vi "EventStream-GetPhotonInfo.vi"() -> ()   [LabVIEW 2023]
doc: "This example demonstrates how to use the Becker&Hickl LabVIEW wrapper VIs to acquire a decay curve using the FIFO Stream mode.\nA measurement is stopped either when accumulating the desired number of photons or the collection time expired.\nThe SPC parameters can be adjusted during the run. The rates and status flags are continuously updated.\nThis VI is based on the C-example part 5 in use_spcm.c\n\ninfo@becker-hickl.com"
uses:
  SPC_Wrappers/SPC_Controls/Fifo_Type.ctl
  SPC_Wrappers/SPC_Controls/SPC_RatesCluster.ctl
  Example_Controls/UserInput.ctl
  Example_Controls/FIFOStream_States.ctl
  SPC_Wrappers/SPC_Controls/SPC_PhotInfo64.ctl
  SPC_Wrappers/SPC_Controls/StateCluster.ctl
  SPC_Wrappers/SPC_Controls/par_id.ctl
  SPC_Wrappers/SPC_Controls/WhatToRead.ctl
  <vilib>/Utility/miscctls.llb/LVTextColorsTypeDef.ctl
panel:
  out "Photon Count reached":bool
  out "SPC_StateCluster":T1
  out "Col.TimerExpired":bool
  out "FlagEvents":i32[](array[numeric])
  out "MTDivider":i32
  in  "BinningResolution [ms]":dbl=5.0 format="%^#_6g"
  out "Current Time":dbl format="%.2g"
  out "No of Read Photons":u64 caption="No of Read\nPhotons"
  out "Current Offset in Stream":u64 caption="Current Offset\nin Stream"
  out "Stream Size":u64
  out "StreamHandle":i16
  in  "Photons to Count":i32=200000
  out "PhotonCount":i32
  out "PhotInfo64":T2[](array[typedef]) {"flags" max=3 format="%016b"; "rout_chan" step=1; "micro_time" step=1; "mtime" step=1}
  out "MCS TimeLine":u64[](graph)=[53, 53, 49, 54, 54, 56, 60, 46, 54, 56, 58, 41, 54, 61, 59, 67, 51, 63, 53, 53, 67, 47, 57, 51, 50, 50, 53, 49, 58, 49, 49, 61, 51, 71, 69, 51, 67, 62, 73, 44, 51, 56, 52, 66, 53, 54, 41, 59, 53, 51, 44, 68, 59, 46, 56, 48, 48, 54, 55, 62, 60, 54, 51, 48, 49, 53, 65, 66, 74, 64, 51, 55, 54, 40, 37, 64, 54, 54, 49, 51, 45, 49, 56, 50, 48, 52, 77, 60, 52, 52, 57, 53, 59, 68, 42, 55, 54, 47, 59, 56, 49, 53, 46, 51, 49, 51, 61, 45, 53, 58, 49, 42, 54, 50, 48, 54, 47, 40, 66, 50, 49, 41, 51, 46, 56, 49, 58, 67, 50, 63, 57, 55, 45, 62, 54, 42, 56, 57, 55, 50, 52, 53, 40, 46, 64, 52, 46, 47, 53, 49, 61, 50, 64, 72, 61, 54, 48, 46, 60, 41, 55, 67, 59, 50, 59, 64, 58, 55, 56, 69, 44, 56, 46, 64, 49, 44, 56, 46, 60, 56, 46, 57, 48, 45, 51, 77, 57, 48, 58, 54, 42, 56, 49, 58, 54, 46, 58, 47, 66, 51, 70, 45, 50, 39, 50, 52, 58, 59, 63, 39, 47, 47, 53, 53, 60, 63, 72, 48, 49, 41, 49, 43, 44, 53, 44, 48, 72, 47, 74, 54, 51, 42, 52, 66, 40, 66, 62, 40, 61, 36, 54, 59, 56, 64, 48, 50, 65, 49, 61, 51, 50, 56, 57, 41, 48, 48, 61, 49, 67, 40, 50, 50, 53, 43, 52, 60, 64, 42, 52, 52, 63, 50, 47, 66, 45, 49, 47, 57, 58, 52, 65, 65, 50, 58, 57, 66, 56, 47, 51, 51, 59, 62, 60, 53, 63, 61, 65, 71, 47, 57, 59, 37, 44, 54, 59, 49, 51, 55, 57, 40, 49, 52, 42, 56, 64, 53, 47, 40, 69, 48, 53, 54, 49, 38, 49, 49, 55, 60, 45, 45, 52, 68, 52, 52, 52, 60, 57, 46, 43, 62, 62, 53, 59, 49, 48, 61, 51, 43, 58, 49, 44, 58, 54, 59, 59, 49, 60, 52, 55, 51, 46, 55, 53, 54, 63, 50, 51, 47, 57, 53, 59, 38, 48, 58, 56, 41, 51, 36, 68, 77, 53, 56, 52, 58, 43, 60, 70, 52, 57, 60, 45, 50, 57, 46, 44, 44, 47, 51, 48, 49, 47, 51, 55, 63, 57, 65, 39, 59, 39, 55, 52, 46, 57, 48, 56, 60, 46, 46, 63, 59, 45, 41, 61, 56, 50, 51, 46, 50, 48, 49, 52, 50, 43, 49, 43, 56, 44, 49, 53, 47, 54, 52, 57, 46, 49, 49, 62, 47, 54, 51, 54, 59, 62, 36, 49, 50, 42, 69, 58, 55, 63, 38, 65, 47, 46, 67, 51, 53, 68, 57, 61, 43, 53, 42, 55, 60, 59, 56, 51, 55, 47, 55, 48, 47, 40, 57, 53, 60, 54, 51, 56, 57, 55, 57, 62, 41, 58, 59, 67, 60, 62, 49, 59, 56, 50, 63, 41, 51, 53, 53, 56, 63, 53, 46, 50, 50, 60, 49, 71, 51, 52, 58, 43, 47, 59, 69, 50, 57, 58, 66, 66, 54, 51, 63, 52, 54, 53, 44, 54, 49, 52, 57, 46, 53, 49, 63, 68, 55, 53, 49, 43, 57, 53, 62, 53, 49, 55, 57, 54, 56, 58, 53, 64, 62, 63, 62, 48, 55, 49, 55, 54, 42, 51, 57, 50, 58, 46, 56, 42, 57, 53, 65, 60, 47, 61, 69, 58, 53, 54, 47, 49, 45, 66, 52, 51, 52, 55, 52, 51, 43, 51, 55, 59, 60, 57, 63, 65, 47, 55, 36, 54, 42, 54, 56, 49, 43, 41, 51, 57, 59, 57, 63, 54, 48, 42, 62, 61, 64, 43, 43, 49, 58, 61, 59, 53, 61, 52, 52, 56, 52, 61, 60, 52, 51, 60, 45, 58, 56, 54, 68, 51, 42, 52, 59, 53, 48, 48, 61, 53, 52, 51, 60, 55, 53, 62, 60, 52, 49, 50, 47, 61, 48, 52, 52, 55, 51, 55, 40, 52, 65, 56, 53, 57, 47, 59, 55, 60, 50, 56, 54, 62, 45, 47, 38, 61, 50, 56, 51, 47, 50, 62, 63, 53, 55, 59, 48, 57, 53, 65, 48, 50, 54, 52, 56, 56, 56, 60, 61, 61, 57, 47, 51, 68, 48, 62, 49, 60, 66, 57, 72, 53, 56, 45, 50, 56, 52, 61, 55, 63, 50, 57, 49, 68, 49, 55, 70, 55, 48, 48, 47, 47, 60, 60, 55, 60, 46, 49, 44, 53, 64, 54, 58, 63, 49, 55, 64, 49, 46, 61, 60, 62, 53, 49, 56, 56, 53, 50, 58, 48, 60, 73, 61, 52, 62, 47, 53, 54, 47, 53, 46, 57, 63, 50, 60, 47, 69, 41, 46, 58, 56, 54, 60, 53, 64, 49, 69, 63, 57, 42, 55, 60, 56, 61, 54, 73, 58, 71, 34, 40, 59, 54, 60, 51, 59, 64, 55, 63, 59, 59, 51, 52, 39, 49, 41, 57, 49, 50, 50, 59, 54, 38, 55, 65, 50, 53, 66, 48, 67, 48, 57, 52, 46, 58, 55, 65, 58, 45, 48, 53, 42, 50, 51, 61, 56, 58, 64, 57, 47, 58, 49, 53, 51, 49, 52, 56, 45, 51, 50, 54, 52, 56, 48, 52, 63, 54, 61, 55, 53, 53, 51, 48, 61, 54, 56, 52, 48, 68, 61, 51, 55, 69, 43, 65, 53, 67, 63, 62, 53, 40, 56, 37, 48, 65, 51, 48, 47, 54, 57, 41, 39, 52, 52, 46, 57, 62, 52, 50, 59, 65, 49, 59, 50, 56, 60, 46, 50, 65, 62, 59, 51, 49, 52, 74, 62, 62, 53, 59, 56, 46, 43, 68, 50, 53, 52, 66, 48, 51, 58, 51, 59, 51, 65, 78, 41, 44, 68, 56, 42, 66, 51, 47, 55, 43, 59, 53, 49, 49, 64, 55, 53, 58, 58, 45, 53, 58, 47, 57, 53, 61, 59, 64, 46, 62, 64, 60, 48, 51, 65, 53, 50]
  out "EventCount":u32
  out "State":T3
  out "SPC_RatesCluster":T4={"Sync"=49999104.0, "CFD"=298560.0, "TAC"=288832.0, "ADC"=255952.0} {"Sync" scale=0.0..6000000.0; "ADC" scale=0.0..1000000.0; "TAC" scale=0.0..1000000.0; "CFD" scale=0.0..1000000.0}
  out "MT clock [ns]":dbl=25.0
  out "Fifo Type":T5=7 items=["48 bits SPC-6x0"=2, "32 bits SPC-6x0"=3, "32 bits SPC-130"=4, "32 bits SPC-830"=5, "32 bits SPC-140"=6, "32 bits SPC-150\\160\\180"=7, "32 bits DPC-230"=8, "32 bits FIFO_IMAGE"=9, "FIFO_D590"=10, "FIFO_TDC"=11, "FIFO_TDC_ABS"=12]
  in  "Stop":bool
  in  "Start Meas":bool
  in  "User Input":T6={"tac_range"=50.033573, "tac_gain"=3, "tac_offset"=10.0, "tac_limit_high"=100.0, "tac_limit_low"=0.0, "collect_time"=5.0, "sync_threshold"=-70.588234, "sync_zc_level"=-5.2913384, "sync_freq_div"=1, "cfd_limit_low"=-50.980392, "cfd_zc_level"=5.2913384} {"sync_freq_div" items=["1"=1, "2"=2, "4"=4]; "cfd_zc_level" min=-96 max=96 step=0.1 format="%#_3g"; "cfd_limit_low" min=-500 max=0 step=0.1 format="%#_3g"; "sync_zc_level" min=-96 max=96 step=0.1 format="%#_3g"; "sync_threshold" min=-500 max=-20 step=0.1 format="%#_3g"; "tac_limit_low" format="%.3g"; "tac_limit_high" min=0 max=100 step=0.1 format="%.3g"; "collect_time" min=1e-07 max=100000 step=0.001; "tac_offset" min=0 max=100 step=0.1 format="%.4g"; "tac_gain" min=1 max=15 step=1; "tac_range" format="%^#_6g"}
  out "Decay":i32[](graph)=[0, 0, 0, 0, 0, 0, 0, 0, 0, 0, 0, 0, 0, 0, 0, 0, 0, 0, 0, 0, 0, 0, 0, 0, 0, 0, 0, 0, 0, 0, 0, 0, 0, 0, 0, 0, 0, 0, 0, 0, 0, 0, 0, 0, 0, 0, 0, 0, 0, 0, 0, 0, 0, 0, 0, 0, 0, 0, 0, 0, 0, 0, 0, 0, 0, 0, 0, 0, 0, 0, 0, 0, 0, 0, 0, 0, 0, 0, 0, 0, 0, 0, 0, 0, 0, 0, 0, 0, 0, 0, 0, 0, 0, 0, 0, 0, 0, 0, 0, 0, 0, 0, 0, 0, 0, 0, 0, 0, 0, 0, 0, 0, 0, 0, 0, 0, 0, 0, 0, 0, 0, 0, 0, 0, 0, 0, 0, 0, 0, 0, 0, 0, 0, 0, 0, 0, 0, 0, 0, 0, 0, 0, 0, 0, 0, 0, 0, 0, 0, 0, 0, 0, 0, 0, 0, 0, 0, 0, 0, 0, 0, 0, 0, 0, 0, 0, 0, 0, 0, 0, 0, 0, 0, 0, 0, 0, 0, 0, 0, 0, 0, 0, 0, 0, 0, 0, 0, 0, 0, 0, 0, 0, 0, 0, 0, 0, 0, 0, 0, 0, 0, 0, 0, 0, 0, 0, 0, 0, 0, 0, 0, 0, 0, 0, 0, 0, 0, 0, 0, 0, 0, 0, 0, 0, 0, 0, 0, 0, 0, 0, 0, 0, 0, 0, 0, 0, 0, 0, 0, 0, 0, 0, 0, 0, 0, 0, 0, 0, 0, 0, 0, 0, 0, 0, 0, 0, 0, 0, 0, 0, 0, 0, 0, 0, 0, 0, 0, 0, 0, 0, 0, 0, 0, 0, 0, 0, 0, 0, 0, 0, 0, 0, 0, 0, 0, 0, 0, 0, 0, 0, 0, 0, 0, 0, 0, 0, 0, 0, 0, 0, 0, 0, 0, 0, 0, 0, 0, 0, 0, 0, 0, 0, 0, 0, 0, 0, 0, 0, 0, 0, 0, 0, 0, 0, 0, 0, 0, 0, 0, 0, 0, 0, 0, 0, 0, 0, 0, 0, 0, 0, 0, 0, 0, 0, 0, 0, 0, 0, 0, 0, 0, 0, 0, 0, 0, 0, 0, 0, 0, 0, 0, 0, 0, 0, 0, 0, 0, 0, 0, 0, 0, 0, 0, 0, 0, 0, 0, 0, 0, 0, 0, 0, 0, 0, 0, 0, 0, 0, 0, 0, 0, 0, 0, 0, 0, 0, 0, 0, 0, 0, 0, 0, 0, 0, 0, 0, 0, 0, 0, 0, 0, 0, 0, 0, 0, 0, 0, 0, 0, 0, 0, 0, 0, 0, 0, 0, 0, 0, 0, 0, 0, 0, 0, 0, 0, 0, 0, 0, 0, 0, 0, 0, 0, 0, 0, 0, 0, 0, 0, 0, 0, 0, 0, 0, 0, 0, 0, 0, 0, 0, 0, 0, 0, 0, 0, 0, 0, 0, 0, 0, 0, 0, 0, 0, 0, 0, 0, 0, 0, 0, 0, 0, 0, 0, 0, 0, 0, 0, 0, 0, 0, 0, 0, 0, 0, 0, 0, 0, 0, 0, 0, 0, 0, 0, 0, 0, 0, 0, 0, 0, 0, 0, 0, 0, 0, 0, 0, 0, 0, 0, 0, 0, 0, 0, 0, 0, 0, 0, 0, 0, 0, 0, 0, 0, 0, 0, 0, 0, 0, 0, 0, 0, 0, 0, 0, 0, 0, 0, 0, 0, 0, 0, 0, 0, 0, 0, 0, 0, 0, 0, 0, 0, 0, 0, 0, 0, 0, 0, 0, 0, 0, 0, 0, 0, 0, 0, 0, 0, 0, 0, 0, 0, 0, 0, 0, 0, 0, 0, 0, 0, 0, 0, 0, 0, 0, 0, 0, 0, 0, 0, 0, 0, 0, 0, 0, 0, 0, 0, 0, 0, 0, 0, 0, 0, 0, 0, 0, 0, 0, 0, 0, 0, 0, 0, 0, 0, 0, 0, 0, 0, 0, 0, 0, 0, 0, 0, 0, 0, 0, 0, 0, 0, 0, 0, 0, 0, 0, 0, 0, 0, 0, 0, 0, 0, 0, 0, 0, 0, 0, 0, 0, 0, 0, 0, 0, 0, 0, 0, 0, 0, 0, 0, 0, 0, 0, 0, 0, 0, 0, 0, 0, 0, 0, 0, 0, 0, 0, 0, 0, 0, 0, 0, 0, 0, 0, 0, 0, 0, 0, 0, 0, 0, 0, 0, 0, 0, 0, 0, 0, 0, 0, 0, 0, 0, 0, 0, 0, 0, 0, 0, 0, 0, 0, 0, 0, 0, 0, 0, 0, 0, 0, 0, 0, 0, 0, 0, 0, 0, 0, 0, 0, 0, 0, 0, 0, 0, 0, 0, 0, 0, 0, 0, 0, 0, 0, 0, 0, 0, 0, 0, 0, 0, 0, 0, 0, 0, 0, 0, 0, 0, 0, 0, 0, 0, 0, 0, 0, 0, 0, 0, 0, 0, 0, 0, 0, 0, 0, 0, 0, 0, 0, 0, 0, 0, 0, 0, 0, 0, 0, 0, 0, 0, 0, 0, 0, 0, 0, 0, 0, 0, 0, 0, 0, 0, 0, 0, 0, 0, 0, 0, 0, 0, 0, 0, 0, 0, 0, 0, 0, 0, 0, 0, 0, 0, 0, 0, 0, 0, 0, 0, 0, 0, 0, 0, 0, 0, 0, 0, 0, 0, 0, 0, 0, 0, 0, 0, 0, 0, 0, 0, 0, 0, 0, 0, 0, 0, 0, 0, 0, 0, 0, 0, 0, 0, 0, 0, 0, 0, 0, 0, 0, 0, 0, 0, 0, 0, 0, 0, 0, 0, 0, 0, 0, 0, 0, 0, 0, 0, 0, 0, 0, 0, 0, 0, 0, 0, 0, 0, 0, 0, 0, 0, 0, 0, 0, 0, 0, 0, 0, 0, 0, 0, 0, 0, 0, 0, 0, 0, 0, 0, 0, 0, 0, 0, 0, 0, 0, 0, 0, 0, 0, 0, 0, 0, 0, 0, 0, 0, 0, 0, 0, 0, 0, 0, 0, 0, 0, 0, 0, 0, 0, 0, 0, 0, 0, 0, 0, 0, 0, 0, 0, 0, 0, 0, 0, 0, 0, 0, 0, 0, 0, 0, 0, 0, 0, 0, 0, 1, 0, 2, 0, 3, 1, 1, 1, 4, 2, 3, 11, 3, 4, 7, 5, 6, 4, 2, 7, 7, 8, 7, 8, 10, 6, 8, 8, 3, 6, 3, 3, 3, 5, 4, 5, 0, 5, 4, 5, 5, 3, 8, 5, 5, 4, 3, 1, 4, 6, 7, 6, 7, 8, 9, 6, 2, 5, 7, 4, 7, 4, 6, 5, 5, 12, 5, 4, 5, 10, 4, 6, 5, 7, 8, 3, 6, 5, 7, 5, 9, 2, 3, 9, 4, 5, 5, 5, 4, 9, 7, 6, 8, 2, 5, 3, 9, 3, 7, 4, 7, 2, 6, 5, 4, 6, 8, 4, 2, 7, 4, 4, 7, 2, 6, 6, 2, 9, 3, 5, 8, 6, 4, 7, 7, 9, 5, 5, 6, 4, 3, 7, 5, 4, 9, 6, 4, 1, 7, 9, 4, 4, 3, 10, 7, 5, 13, 10, 11, 8, 2, 5, 3, 3, 4, 7, 4, 5, 6, 8, 3, 3, 10, 5, 6, 5, 3, 9, 1, 9, 5, 4, 5, 3, 2, 4, 5, 4, 3, 3, 5, 3, 7, 4, 8, 6, 8, 11, 17, 10, 16, 15, 28, 20, 33, 22, 22, 26, 30, 33, 28, 27, 36, 31, 40, 40, 45, 38, 41, 57, 51, 42, 46, 56, 51, 59, 45, 51, 60, 59, 53, 48, 60, 53, 58, 49, 68, 57, 54, 64, 60, 61, 61, 67, 68, 68, 52, 60, 73, 71, 88, 61, 67, 82, 63, 74, 72, 80, 83, 78, 96, 87, 67, 80, 65, 77, 74, 77, 75, 60, 65, 89, 85, 88, 95, 80, 70, 66, 81, 84, 83, 78, 82, 80, 83, 84, 87, 80, 74, 60, 94, 90, 94, 96, 79, 88, 77, 73, 89, 73, 86, 79, 77, 85, 75, 68, 88, 84, 63, 62, 76, 70, 72, 74, 80, 80, 80, 72, 75, 73, 74, 82, 86, 102, 88, 91, 63, 84, 67, 77, 64, 72, 83, 73, 78, 75, 71, 71, 74, 70, 67, 58, 63, 76, 63, 70, 70, 62, 74, 82, 60, 64, 64, 65, 66, 67, 74, 70, 62, 84, 72, 66, 60, 73, 55, 72, 80, 54, 68, 80, 56, 59, 65, 48, 64, 61, 52, 60, 78, 60, 56, 71, 51, 53, 50, 55, 61, 45, 54, 52, 57, 61, 62, 60, 58, 60, 58, 50, 60, 50, 61, 64, 69, 50, 54, 51, 45, 61, 49, 46, 59, 42, 39, 48, 52, 55, 55, 56, 56, 59, 57, 63, 60, 54, 52, 46, 50, 54, 60, 45, 45, 43, 59, 52, 40, 53, 54, 48, 57, 46, 48, 68, 55, 44, 43, 48, 36, 53, 59, 42, 49, 43, 59, 38, 50, 44, 51, 61, 54, 44, 46, 39, 47, 48, 54, 38, 54, 54, 59, 43, 59, 48, 42, 50, 31, 53, 45, 46, 40, 41, 52, 52, 45, 38, 45, 50, 38, 47, 50, 44, 41, 36, 45, 39, 41, 53, 39, 63, 46, 52, 36, 34, 41, 52, 52, 56, 44, 58, 43, 39, 35, 42, 38, 46, 46, 37, 44, 34, 55, 38, 40, 39, 38, 40, 35, 58, 43, 42, 56, 47, 36, 35, 36, 40, 46, 45, 40, 41, 45, 35, 25, 47, 30, 38, 38, 46, 41, 33, 38, 43, 40, 42, 26, 39, 32, 43, 39, 34, 38, 35, 38, 49, 34, 36, 27, 43, 31, 47, 35, 44, 41, 26, 30, 33, 35, 31, 37, 26, 39, 27, 32, 27, 44, 35, 40, 43, 45, 44, 32, 35, 37, 40, 38, 34, 24, 40, 33, 37, 29, 27, 22, 37, 45, 35, 31, 36, 29, 20, 40, 37, 34, 35, 31, 37, 24, 31, 33, 30, 32, 25, 31, 33, 35, 28, 33, 38, 34, 32, 35, 30, 33, 33, 31, 33, 27, 40, 32, 23, 33, 39, 28, 40, 30, 36, 22, 26, 27, 31, 31, 40, 32, 27, 18, 30, 37, 29, 31, 44, 44, 35, 29, 33, 30, 34, 40, 37, 30, 19, 26, 32, 31, 32, 33, 27, 28, 37, 41, 27, 29, 21, 30, 34, 31, 30, 25, 25, 30, 27, 25, 25, 34, 33, 19, 25, 30, 32, 29, 32, 34, 30, 32, 21, 31, 27, 34, 30, 40, 30, 28, 38, 35, 30, 21, 21, 26, 28, 25, 21, 37, 23, 30, 36, 34, 24, 36, 36, 19, 17, 27, 19, 32, 29, 27, 21, 33, 22, 23, 30, 23, 31, 22, 27, 35, 23, 19, 27, 30, 34, 32, 32, 27, 36, 28, 35, 24, 30, 27, 21, 23, 16, 23, 28, 22, 29, 19, 21, 19, 30, 29, 26, 18, 30, 34, 31, 25, 22, 35, 15, 27, 31, 26, 28, 26, 24, 34, 23, 23, 18, 34, 28, 19, 27, 21, 15, 27, 24, 24, 18, 19, 20, 23, 25, 36, 28, 19, 24, 27, 24, 20, 25, 12, 15, 24, 21, 31, 27, 25, 26, 38, 27, 18, 23, 20, 18, 29, 17, 24, 26, 19, 20, 15, 22, 26, 21, 16, 25, 22, 23, 29, 24, 26, 15, 19, 25, 25, 22, 20, 25, 18, 24, 20, 21, 27, 20, 28, 26, 21, 21, 25, 23, 24, 25, 25, 17, 26, 32, 18, 28, 30, 25, 14, 20, 26, 23, 34, 14, 23, 26, 19, 19, 21, 23, 27, 20, 32, 23, 15, 29, 27, 22, 28, 19, 26, 24, 18, 22, 18, 27, 25, 23, 25, 21, 26, 25, 33, 24, 24, 26, 15, 17, 24, 19, 25, 35, 18, 26, 27, 20, 12, 18, 28, 24, 23, 21, 21, 23, 20, 16, 22, 21, 13, 23, 19, 22, 21, 16, 18, 23, 24, 20, 27, 14, 23, 23, 20, 19, 15, 30, 10, 17, 21, 15, 28, 17, 16, 20, 24, 16, 21, 18, 22, 18, 20, 19, 24, 17, 24, 19, 15, 36, 18, 27, 16, 16, 19, 17, 22, 24, 19, 20, 23, 17, 23, 18, 14, 27, 23, 17, 19, 17, 22, 22, 19, 17, 23, 22, 21, 18, 8, 28, 23, 17, 15, 27, 15, 15, 22, 16, 20, 21, 24, 16, 18, 22, 19, 18, 21, 20, 20, 22, 28, 17, 13, 24, 10, 17, 18, 6, 28, 20, 11, 21, 27, 19, 20, 23, 16, 17, 19, 20, 18, 22, 22, 13, 20, 11, 11, 21, 22, 17, 23, 21, 8, 16, 22, 20, 20, 15, 14, 14, 17, 26, 13, 19, 13, 17, 13, 14, 10, 13, 21, 12, 16, 23, 12, 17, 19, 13, 16, 12, 10, 16, 15, 15, 20, 18, 21, 19, 17, 18, 19, 23, 22, 6, 10, 17, 28, 18, 12, 10, 18, 12, 18, 13, 15, 13, 19, 18, 16, 14, 23, 19, 22, 22, 18, 7, 20, 16, 18, 19, 14, 17, 21, 13, 18, 20, 16, 26, 21, 14, 16, 16, 14, 22, 20, 10, 14, 23, 10, 17, 19, 13, 23, 14, 19, 20, 15, 14, 18, 13, 14, 16, 20, 22, 17, 12, 14, 14, 21, 10, 9, 15, 12, 17, 12, 13, 9, 17, 20, 15, 17, 16, 22, 16, 7, 24, 18, 20, 14, 17, 11, 19, 12, 13, 17, 19, 14, 11, 17, 16, 15, 12, 17, 18, 18, 14, 12, 17, 18, 21, 16, 16, 18, 11, 17, 11, 16, 22, 15, 11, 11, 24, 24, 16, 21, 18, 21, 16, 10, 15, 20, 14, 15, 18, 9, 11, 20, 18, 6, 21, 18, 18, 12, 17, 22, 16, 18, 16, 16, 11, 10, 12, 17, 11, 14, 26, 12, 13, 13, 12, 15, 16, 12, 15, 18, 13, 18, 22, 16, 17, 13, 17, 20, 14, 22, 13, 16, 19, 10, 11, 12, 10, 22, 28, 19, 17, 14, 14, 9, 11, 10, 17, 15, 11, 18, 11, 16, 13, 13, 6, 14, 11, 11, 15, 8, 18, 14, 18, 11, 15, 5, 14, 21, 11, 17, 17, 19, 16, 10, 13, 10, 14, 14, 17, 14, 18, 16, 18, 15, 20, 7, 13, 13, 11, 11, 14, 10, 11, 17, 7, 23, 20, 21, 10, 14, 16, 18, 20, 7, 19, 10, 19, 14, 9, 14, 10, 15, 11, 19, 18, 15, 10, 12, 10, 14, 13, 11, 7, 13, 17, 12, 16, 4, 15, 8, 21, 14, 13, 19, 21, 21, 7, 15, 14, 13, 15, 13, 16, 20, 15, 7, 10, 17, 23, 3, 10, 12, 11, 11, 15, 15, 10, 23, 12, 15, 18, 9, 12, 9, 7, 10, 12, 14, 9, 11, 13, 12, 19, 10, 12, 17, 12, 18, 12, 12, 15, 8, 13, 10, 13, 12, 14, 12, 9, 16, 11, 9, 17, 12, 9, 9, 11, 13, 7, 8, 16, 10, 16, 12, 8, 14, 13, 16, 13, 8, 10, 9, 13, 11, 13, 6, 16, 18, 16, 14, 13, 12, 9, 11, 12, 14, 12, 10, 12, 14, 10, 13, 13, 12, 18, 11, 17, 14, 10, 13, 7, 14, 14, 10, 13, 7, 8, 16, 13, 12, 12, 11, 12, 10, 15, 13, 9, 7, 8, 10, 17, 10, 13, 11, 18, 16, 18, 15, 8, 13, 12, 8, 10, 11, 14, 15, 14, 10, 9, 14, 10, 10, 9, 12, 8, 10, 5, 17, 14, 11, 9, 12, 9, 17, 10, 9, 12, 9, 15, 15, 12, 10, 14, 13, 9, 10, 13, 8, 7, 14, 8, 13, 16, 18, 9, 11, 8, 14, 14, 13, 9, 12, 13, 16, 8, 8, 9, 11, 13, 12, 11, 10, 13, 17, 9, 10, 13, 12, 11, 6, 16, 9, 6, 17, 6, 11, 10, 11, 12, 11, 14, 11, 8, 10, 16, 13, 11, 11, 12, 13, 9, 6, 6, 13, 6, 9, 7, 14, 8, 7, 12, 12, 12, 10, 10, 6, 19, 5, 13, 10, 16, 9, 10, 10, 8, 10, 9, 15, 9, 12, 11, 8, 14, 11, 7, 9, 9, 11, 6, 9, 12, 14, 11, 11, 11, 12, 14, 13, 8, 10, 14, 12, 12, 10, 9, 14, 8, 12, 16, 9, 15, 12, 16, 17, 13, 10, 11, 8, 13, 5, 6, 19, 13, 13, 22, 10, 11, 8, 10, 12, 9, 6, 7, 14, 8, 11, 9, 12, 15, 12, 11, 13, 6, 10, 11, 12, 8, 10, 11, 11, 7, 10, 11, 10, 12, 8, 6, 8, 9, 7, 9, 9, 9, 9, 8, 14, 13, 10, 11, 11, 9, 12, 9, 12, 13, 6, 10, 4, 11, 7, 9, 9, 15, 16, 5, 8, 8, 11, 15, 5, 10, 20, 7, 4, 8, 6, 13, 15, 9, 13, 13, 12, 6, 14, 7, 9, 11, 10, 11, 13, 11, 11, 6, 6, 10, 9, 9, 8, 11, 8, 10, 15, 12, 17, 10, 10, 8, 10, 7, 16, 7, 13, 10, 16, 10, 8, 8, 14, 11, 6, 14, 6, 13, 5, 8, 4, 14, 7, 10, 9, 6, 6, 9, 8, 13, 11, 13, 10, 15, 9, 12, 13, 3, 10, 7, 9, 7, 9, 10, 8, 10, 7, 10, 11, 9, 15, 8, 13, 17, 11, 5, 11, 7, 4, 18, 10, 13, 9, 6, 5, 5, 13, 9, 15, 10, 14, 8, 6, 8, 12, 7, 9, 10, 14, 9, 10, 13, 10, 12, 10, 11, 8, 8, 8, 12, 7, 11, 10, 9, 10, 14, 17, 11, 14, 12, 4, 14, 9, 7, 8, 4, 7, 12, 10, 8, 7, 15, 14, 5, 14, 12, 14, 11, 13, 7, 11, 10, 9, 7, 2, 4, 8, 7, 7, 12, 10, 11, 11, 10, 7, 15, 10, 11, 8, 8, 7, 11, 11, 11, 8, 7, 10, 8, 14, 3, 15, 7, 10, 8, 4, 11, 8, 9, 8, 5, 7, 8, 11, 13, 7, 12, 5, 12, 13, 14, 10, 3, 9, 13, 10, 14, 8, 11, 12, 11, 11, 7, 11, 15, 11, 5, 17, 12, 7, 6, 5, 7, 6, 6, 12, 10, 12, 8, 6, 12, 12, 11, 10, 9, 7, 9, 12, 7, 11, 15, 9, 15, 9, 10, 4, 13, 12, 8, 7, 10, 13, 11, 6, 10, 10, 10, 10, 7, 10, 9, 11, 9, 10, 8, 11, 9, 5, 7, 7, 8, 9, 7, 9, 11, 9, 7, 10, 6, 15, 11, 8, 11, 7, 9, 12, 14, 13, 8, 10, 7, 8, 7, 6, 13, 5, 6, 5, 8, 5, 8, 12, 11, 10, 8, 6, 8, 8, 13, 7, 4, 8, 4, 9, 7, 9, 9, 11, 11, 14, 11, 5, 7, 7, 6, 6, 6, 5, 7, 6, 5, 4, 9, 7, 13, 3, 13, 12, 12, 12, 8, 9, 7, 5, 6, 8, 11, 6, 10, 12, 4, 7, 7, 10, 9, 7, 10, 5, 13, 11, 8, 6, 13, 10, 17, 8, 7, 14, 9, 16, 5, 6, 7, 11, 10, 2, 12, 6, 5, 6, 14, 7, 9, 11, 5, 5, 11, 5, 6, 9, 9, 6, 2, 8, 7, 9, 10, 7, 7, 6, 6, 10, 4, 7, 4, 11, 10, 8, 4, 10, 5, 10, 8, 5, 6, 6, 12, 13, 7, 6, 10, 16, 10, 10, 10, 6, 8, 3, 8, 6, 12, 8, 5, 10, 5, 10, 7, 7, 8, 11, 7, 11, 6, 7, 6, 8, 14, 11, 9, 8, 6, 3, 8, 8, 7, 11, 5, 8, 7, 10, 8, 9, 13, 9, 10, 6, 11, 1, 6, 7, 6, 8, 18, 11, 9, 7, 7, 5, 8, 8, 7, 4, 15, 14, 7, 13, 2, 5, 5, 11, 10, 5, 9, 8, 5, 11, 6, 5, 11, 6, 11, 9, 7, 3, 10, 10, 15, 5, 9, 8, 4, 8, 8, 10, 9, 7, 6, 12, 11, 11, 8, 13, 14, 3, 5, 13, 8, 6, 9, 11, 5, 12, 6, 10, 9, 3, 8, 15, 9, 12, 7, 5, 7, 7, 7, 10, 10, 10, 13, 8, 5, 7, 8, 2, 6, 5, 11, 9, 13, 5, 12, 11, 8, 11, 9, 5, 10, 2, 8, 7, 5, 7, 9, 4, 7, 16, 8, 6, 7, 8, 7, 7, 6, 11, 12, 6, 8, 6, 6, 6, 8, 6, 11, 10, 11, 7, 9, 6, 12, 7, 7, 3, 10, 4, 4, 5, 8, 12, 9, 6, 8, 9, 9, 12, 9, 10, 9, 10, 5, 4, 10, 8, 10, 6, 10, 5, 7, 6, 7, 7, 7, 5, 10, 3, 4, 8, 7, 7, 13, 10, 4, 17, 11, 5, 2, 10, 7, 2, 10, 7, 12, 10, 7, 8, 8, 8, 12, 13, 5, 11, 11, 7, 3, 7, 14, 7, 7, 6, 10, 5, 8, 7, 5, 4, 5, 8, 7, 8, 11, 8, 10, 5, 7, 8, 2, 7, 4, 3, 7, 8, 7, 9, 8, 5, 7, 8, 9, 4, 6, 5, 2, 6, 3, 13, 9, 5, 7, 5, 11, 10, 4, 10, 3, 14, 2, 8, 6, 3, 16, 7, 12, 7, 6, 5, 9, 4, 8, 9, 6, 7, 8, 10, 6, 11, 14, 9, 9, 6, 9, 7, 10, 9, 10, 6, 8, 7, 10, 6, 7, 10, 6, 7, 3, 7, 9, 3, 10, 8, 8, 8, 7, 4, 12, 10, 5, 10, 11, 5, 8, 11, 9, 7, 9, 4, 4, 7, 7, 8, 8, 7, 10, 3, 11, 6, 7, 4, 7, 11, 6, 5, 8, 7, 7, 6, 7, 11, 6, 11, 6, 15, 5, 9, 10, 9, 1, 6, 5, 6, 6, 4, 7, 11, 6, 6, 8, 9, 5, 12, 10, 3, 7, 9, 7, 10, 5, 8, 9, 5, 8, 13, 3, 5, 7, 8, 7, 5, 7, 8, 9, 10, 5, 7, 9, 4, 9, 6, 4, 9, 5, 6, 9, 9, 3, 6, 5, 5, 4, 4, 9, 6, 11, 5, 9, 5, 9, 7, 4, 8, 9, 7, 5, 8, 9, 12, 8, 6, 6, 8, 9, 8, 7, 8, 4, 7, 10, 7, 7, 8, 8, 11, 10, 3, 8, 7, 5, 8, 12, 6, 9, 9, 7, 5, 10, 8, 10, 6, 7, 10, 10, 5, 7, 7, 6, 4, 3, 8, 9, 11, 8, 4, 10, 11, 5, 4, 7, 9, 7, 10, 6, 4, 5, 3, 4, 8, 6, 5, 6, 6, 8, 9, 4, 3, 9, 10, 5, 7, 7, 4, 8, 10, 5, 11, 8, 8, 11, 11, 5, 11, 5, 6, 6, 5, 4, 6, 8, 6, 5, 4, 10, 7, 4, 6, 6, 6, 7, 10, 4, 4, 5, 13, 8, 11, 4, 5, 12, 9, 5, 5, 7, 5, 12, 7, 6, 4, 7, 7, 3, 4, 5, 7, 8, 7, 2, 4, 9, 8, 7, 5, 8, 8, 8, 8, 4, 8, 6, 9, 9, 6, 3, 8, 5, 5, 5, 4, 5, 7, 5, 8, 5, 1, 4, 7, 7, 5, 7, 5, 8, 8, 6, 4, 4, 5, 7, 5, 6, 5, 10, 11, 6, 4, 9, 7, 8, 5, 5, 11, 6, 7, 3, 14, 9, 6, 8, 7, 5, 6, 7, 6, 4, 5, 3, 8, 7, 5, 5, 5, 6, 9, 9, 7, 8, 9, 11, 5, 5, 5, 6, 7, 8, 10, 7, 5, 5, 9, 5, 7, 5, 8, 6, 6, 2, 5, 11, 9, 7, 5, 7, 6, 8, 7, 8, 2, 8, 3, 5, 10, 6, 5, 9, 7, 9, 5, 9, 7, 9, 7, 9, 16, 4, 10, 3, 8, 5, 10, 5, 7, 3, 7, 8, 5, 12, 8, 4, 7, 5, 9, 7, 7, 7, 7, 3, 7, 7, 10, 4, 5, 11, 8, 14, 7, 8, 5, 9, 8, 8, 10, 6, 9, 5, 5, 9, 9, 6, 4, 11, 1, 6, 6, 5, 7, 3, 7, 9, 5, 10, 3, 5, 9, 11, 0, 8, 10, 6, 7, 5, 6, 8, 15, 4, 4, 7, 8, 10, 6, 7, 5, 2, 3, 6, 3, 2, 9, 5, 2, 6, 6, 6, 6, 5, 1, 6, 7, 4, 9, 6, 5, 6, 7, 11, 7, 2, 7, 6, 6, 6, 9, 7, 10, 8, 10, 6, 2, 6, 6, 3, 9, 6, 11, 6, 3, 4, 5, 4, 7, 8, 4, 3, 8, 5, 6, 4, 6, 8, 5, 8, 7, 5, 4, 7, 8, 3, 11, 7, 6, 6, 6, 5, 5, 11, 13, 4, 9, 2, 4, 8, 4, 8, 9, 5, 5, 5, 7, 3, 4, 7, 9, 3, 8, 6, 9, 6, 3, 9, 9, 6, 7, 8, 6, 10, 8, 4, 3, 7, 7, 3, 8, 5, 9, 3, 4, 8, 9, 5, 3, 9, 4, 6, 3, 4, 3, 7, 4, 3, 6, 7, 1, 3, 6, 8, 1, 11, 2, 0, 7, 2, 6, 5, 5, 8, 7, 5, 3, 6, 5, 3, 9, 3, 3, 5, 11, 5, 2, 8, 5, 5, 3, 5, 5, 6, 5, 1, 2, 3, 3, 3, 5, 3, 2, 1, 5]
  # "This example demonstrates how to use the Becker&Hickl LabVIEW wrapper VIs to acquire a decay curve using the FIFO Stream mode.\nA measurement is stopped either when the desired number of photons is accumulated or the collection time is expired.\nThe User Input parameters can be adjusted during the run. The rates and status flags are continuously updated.\nThis VI is based on the C-example part 5 in use_spcm.c"
  # "StreamInfo"
  # "See Tip-Strip for details"
  # "TAC / Time Range"
  # "CFD"
  # "(start)"
  # "SYNC"
  # "(stop)"
  # "range"
  # "gain"
  # "threshold(LL)"
  # "offset"
  # "limit high"
  # "limit low"
  # "zero cross(ZC)"
  # "Collection Time"
  # "(c) 2022 Becker & Hickl GmbH\n     ALL RIGHTS RESERVED."
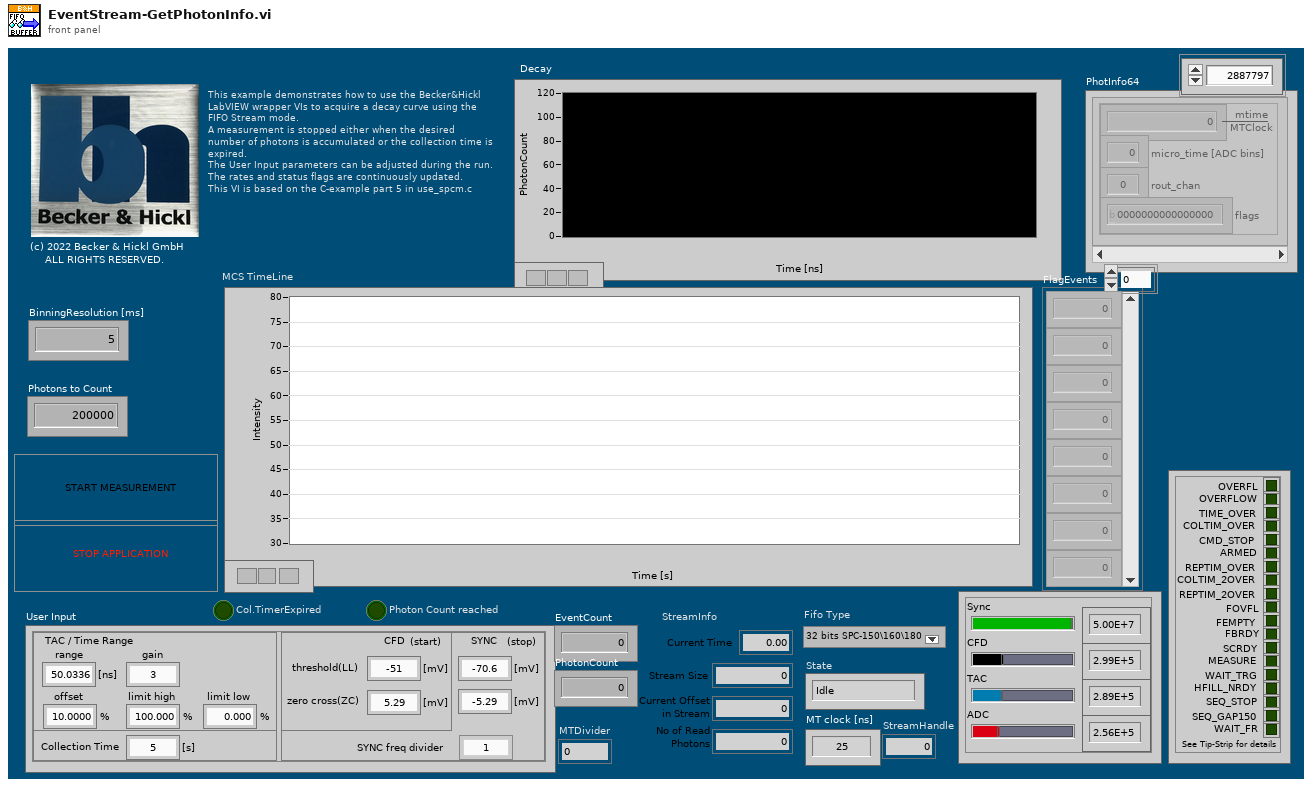
[diagram p1: front panel]
types:
  T1 = typedef "StateCluster.ctl" = cluster{"OVERFL":bool, "OVERFLOW":bool, "TIME_OVER":bool, "COLTIM_OVER":bool, "CMD_STOP":bool, "ARMED":bool, "REPTIM_OVER":bool, "COLTIM_2OVER":bool, "REPTIM_2OVER":bool, "FOVFL":bool, "FEMPTY":bool, "FBRDY":bool, "SCRDY":bool, "MEASURE":bool, "WAIT_TRG":bool, "HFILL_NRDY":bool, "SEQ_STOP":bool, "SEQ_GAP150":bool, "WAIT_FR":bool}
  T2 = typedef "SPC_PhotInfo64.ctl" = cluster{"mtime":u64, "micro_time":u16, "rout_chan":u16, "flags":u16}
  T3 = typedef "FIFOStream_States.ctl" = enum16{"Idle", "PrepareMeas", "TestState", "StopMeas", "ReadFIFO2Stream", "Analyze"}
  T4 = typedef "SPC_RatesCluster.ctl" = cluster{"Sync":sgl, "CFD":sgl, "TAC":sgl, "ADC":sgl}
  T5 = typedef "Fifo_Type.ctl" = i16
  T6 = typedef "UserInput.ctl" = cluster{"tac_range":sgl, "tac_gain":i16, "tac_offset":sgl, "tac_limit_high":sgl, "tac_limit_low":sgl, "collect_time":sgl, "sync_threshold":sgl, "sync_zc_level":sgl, "sync_freq_div":i16, "cfd_limit_low":sgl, "cfd_zc_level":sgl}
  T7 = typedef "SPCModInfo.ctl" = cluster{"Module Type":T8, "Bus Number":i16, "Slot Number":i16, "in Use":i16, "Init Status":i16, "Base I/O Addr":u16}
  T8 = typedef "ModuleType.ctl" = i16
  T9 = typedef "SPCdata.ctl" = cluster{"base_adr":u16, "init":i16, "cfd_limit_low":sgl, "cfd_limit_high":sgl, "cfd_zc_level":sgl, "cfd_holdoff":sgl, "sync_zc_level":sgl, "sync_holdoff":sgl, "sync_threshold":sgl, "tac_range":sgl, "sync_freq_div":i16, "tac_gain":i16, "tac_offset":sgl, "tac_limit_low":sgl, "tac_limit_high":sgl, "adc_resolution":i16, "ext_latch_delay":i16, "collect_time":sgl, "display_time":sgl, "repeat_time":sgl, "stop_on_time":i16, "stop_on_ovfl":i16, "dither_range":i16, "count_incr":i16, "mem_bank":i16, "dead_time_comp":i16, "scan_control":u16, "routing_mode":u16, "tac_enable_hold":sgl, "pci_card_no":i16, "mode":u16, "scan_size_x":u32, "scan_size_y":u32, "scan_rout_x":u32, "scan_rout_y":u32, "scan_flyback":u32, "scan_borders":u32, "scan_polarity":u16, "pixel_clock":u16, "line_compression":u16, "trigger":u16, "pixel_time":sgl, "ext_pixclk_div":u32, "rate_count_time":sgl, "macro_time_clk":i16, "add_select":i16, "test_eep":i16, "adc_zoom":i16, "img_size_x":u32, "img_size_y":u32, "img_rout_x":u32, "img_rout_y":u32, "xy_gain":i16, "master_clock":i16, "adc_sample_delay":i16, "detector_type":i16, "chan_enable":u32, "chan_slope":u32, "chan_spec_no":u32, "tdc_control":u32, "tdc_offset1":sgl, "tdc_offset2":sgl, "tdc_offset3":sgl, "tdc_offset4":sgl, "tdc_offset5":sgl, "tdc_offset6":sgl, "cfd_th5_tdc":sgl, "cfd_th6_tdc":sgl, "cfd_zc5_tdc":sgl, "cfd_zc6_tdc":sgl, "future_reserve1":u64, "future_reserve2":u64, "future_reserve3":u64, "future_reserve4":u64}
  T10 = typedef "LVTextColorsTypeDef.ctl" = cluster{"Text Color":u32, "Background Color":u32}
  T11 = typedef "WhatToRead.ctl" = cluster{"Valid Photons":bool, "Invalid Photons":bool, "Pixel":bool, "Line":bool, "Frame":bool, "Marker 3":bool}
  T12 = cluster{"PhotInfo64":T2[], u64[], i32[], "FlagEvents":i32[]}
  T13 = typedef "par_id.ctl" = i16
  T14 = typedef "SPC_PhotStreamInfo.ctl" = cluster{"FIFO Type":i16, "Stream Type":i16, "Macro Time Clock [0.1ns]":i32, "Routing Channels":i16, "What To Read":i16, "No of Files in Stream":i16, "No of Ready Files":i16, "Stream Base Name":string, "Current FIle Name":string, "1st File Number":i16, "Current File Number":i16, "No of FIFO Overruns":i32, "Stream Size":u64, "Current Offset in Stream":u64, "Offset in Current File":u64, "No of Invalid Photons":u64, "No of Read Photons":u64, "No of Read Markers 0 (Pixel)":u64, "No of Read Markers 1 (Line)":u64, "No of Read Markers 2 (Frame)":u64, "No of Read Markers 3":u64, "Start Offset of 1st Photon (DPC-230 only)":u32, "No of Buffers":i16, "No of Ready Buffers":i16, "Current Buffer Offset":u32, "Start OR Mask":u32, "Start AND Mask":u32, "Stop OR Mask":u32, "Stop AND Mask":u32, "Start Found":i16, "Stop Reached":i16, "Start Time":dbl, "Stop Time":dbl, "Current Time":dbl, "Channels Present When Start Found":u32, "Channels Present When Stop Found":u32}
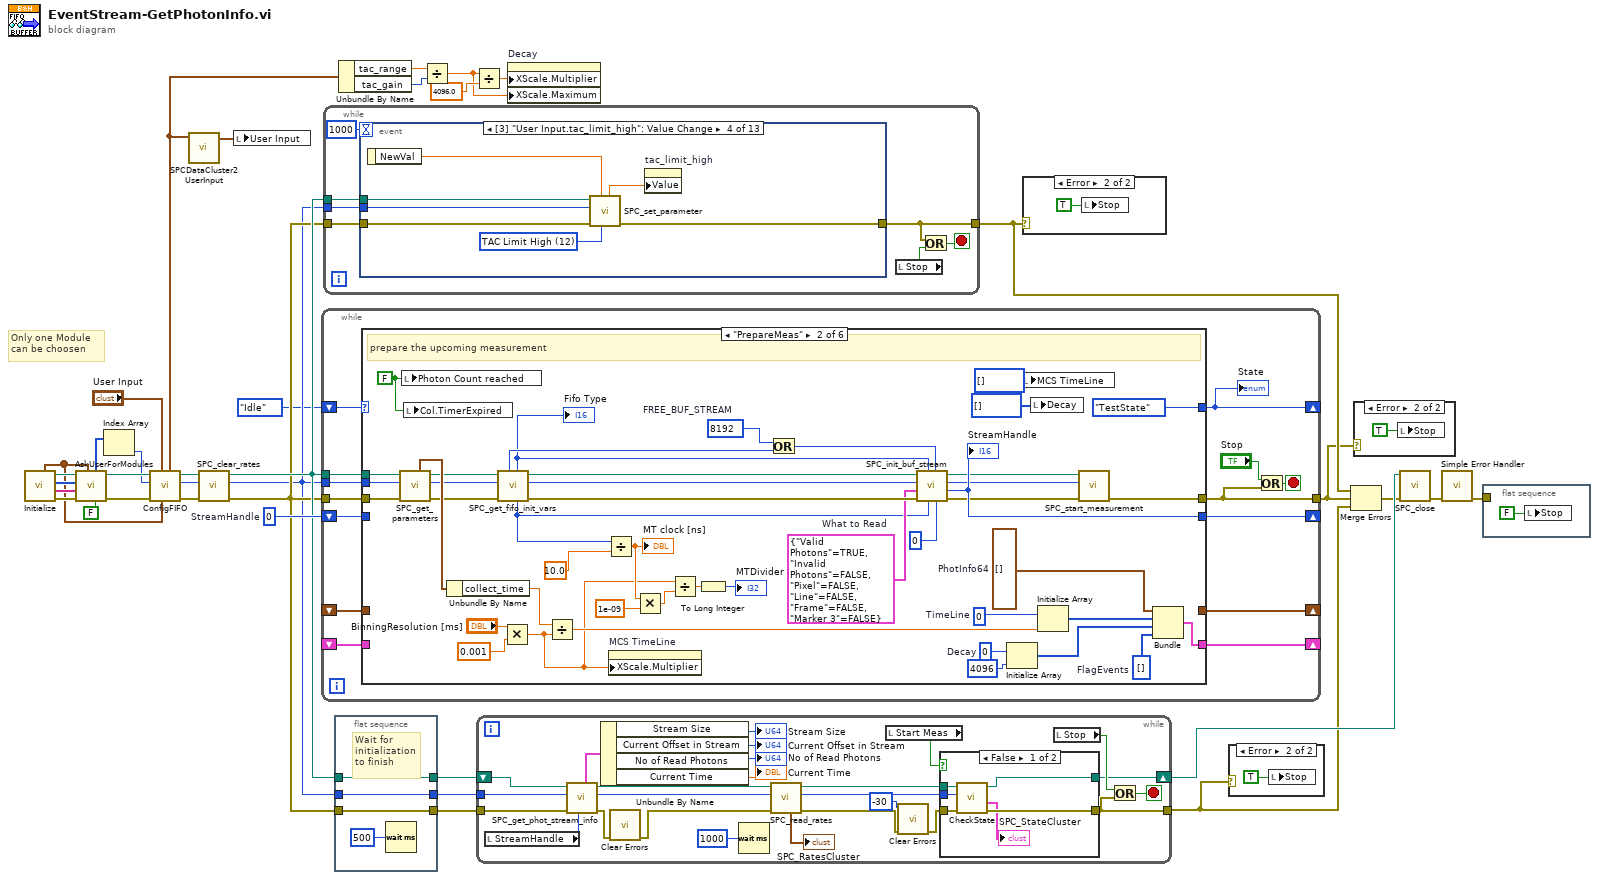
[diagram p0: block diagram]
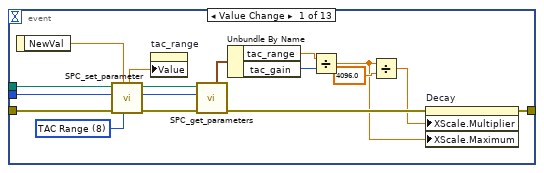
[diagram p2: hidden frame]
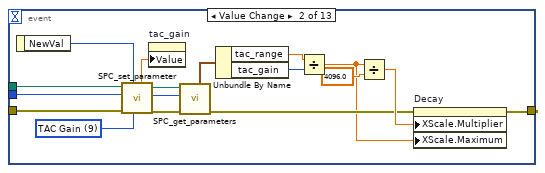
[diagram p3: hidden frame]
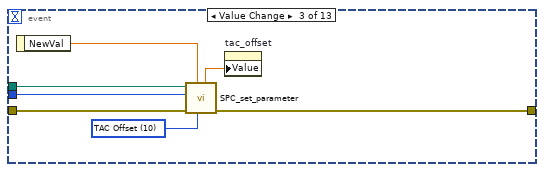
[diagram p4: hidden frame]
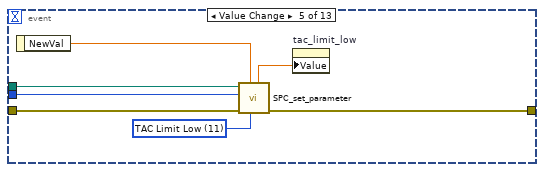
[diagram p5: hidden frame]
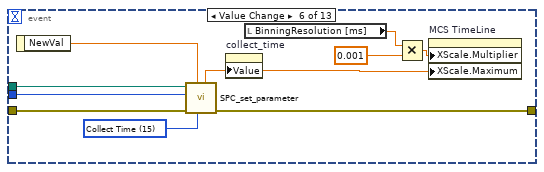
[diagram p6: hidden frame]
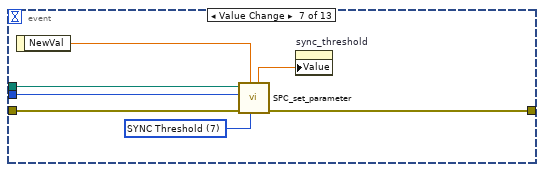
[diagram p7: hidden frame]
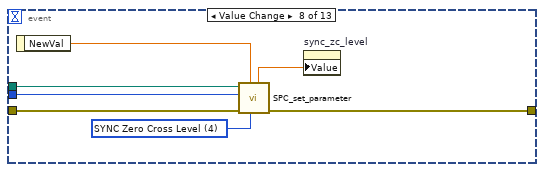
[diagram p8: hidden frame]
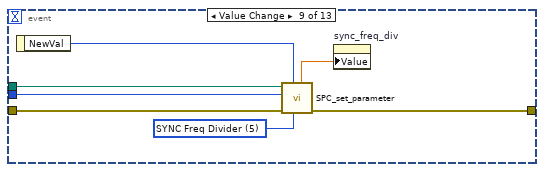
[diagram p9: hidden frame]
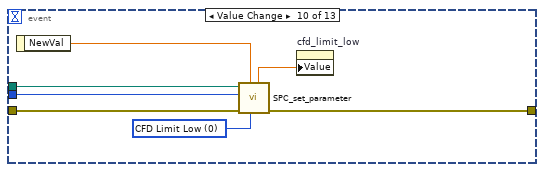
[diagram p10: hidden frame]
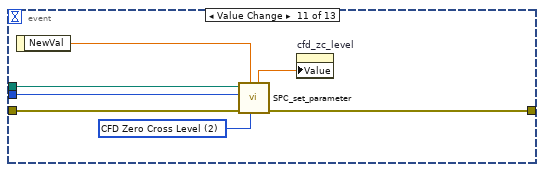
[diagram p11: hidden frame]
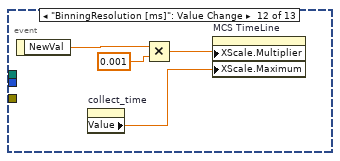
[diagram p12: hidden frame]
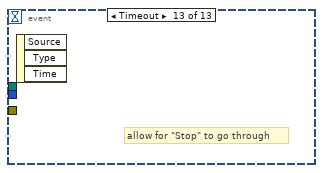
[diagram p13: hidden frame]
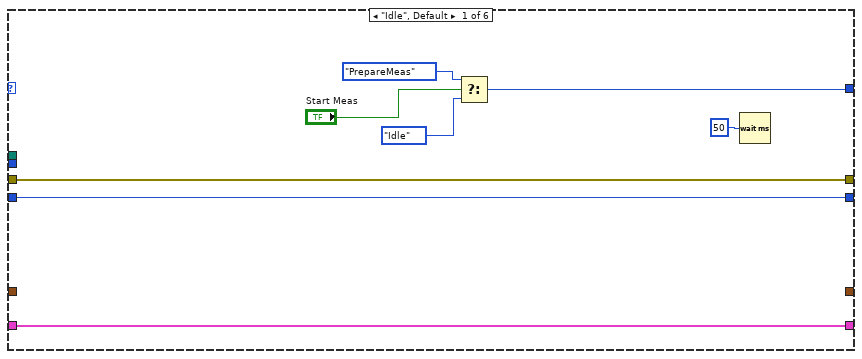
[diagram p14: hidden frame]
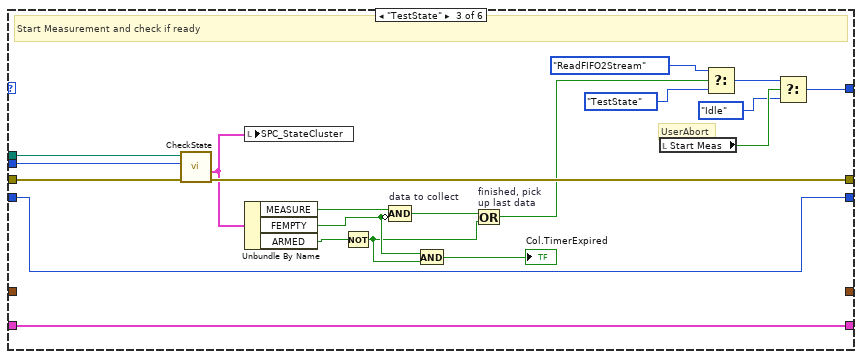
[diagram p15: hidden frame]
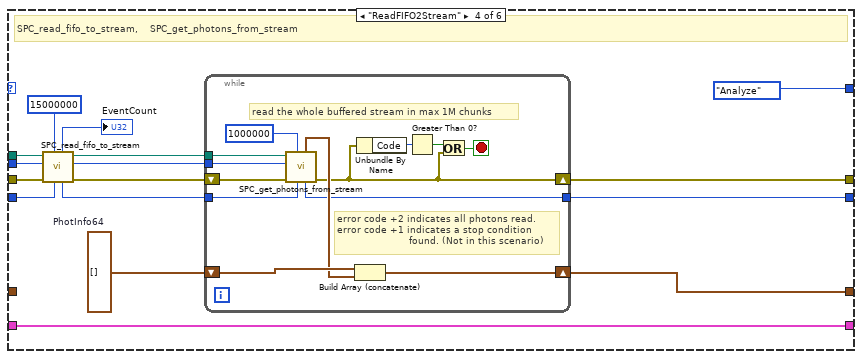
[diagram p16: hidden frame]
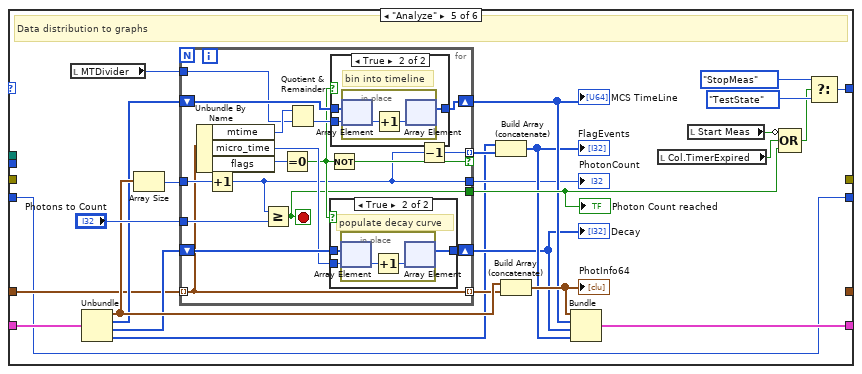
[diagram p17: hidden frame]
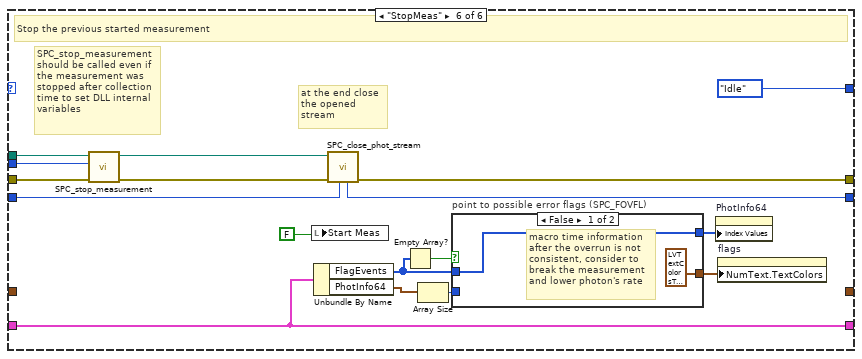
[diagram p20: hidden frame]
diagram:
  w28 = i16 0  # StreamHandle
  # "Only one Module\ncan be choosen"
  n1 = call "Initialize.vi"() -> ("ErrorOut"=w34:errorcluster, "SerialNumbersArray"=w35:string[], "ModuleNoArray"=w29:i16[], "DLL Path"=w33:path, "SPCModulesArray"=w14:T7[])  [unwired: 7 in]
  n2 = call "AskUserForModules.vi"("MultiModule"=FALSE, "SPCModulesArray"=w14, "Error In"=w34, "Serial Number"=w35, "ModuleNoArray"=w29, "DLL Path"=w33) -> ("Error Out"=w5:errorcluster, "DLL Path"=w23:path, "ActiveModuleNo"=w36:i16[])  [unwired: 1 in, 2 out]
  n3 = Index Array(array=w36) -> (element=w22:i16)  [unwired: 1 in]
  n4 = call "ConfigFIFO.vi"("Used Model Array"=w14, "User Input"="User Input", "Error In"=w5, "Module No"=w22, "DLL Path"=w23) -> ("Error Out"=w20:errorcluster, "Module No"=w19:i16, "DLL Path"=w21:path, "SPC Data"=w4:T9)  [unwired: 3 in]
  n5 = call "SPCDataCluster2UserInput.vi"("SPCdata In"=w4) -> ("UserInput Out"=w3:T6)  [unwired: 10 in]
  n6 = call "SPC_clear_rates.vi"("Error In"=w20, "Module no"=w19, "DLL Path"=w21) -> ("Error Out"=w17:errorcluster, "Module  No"=w16:i16, "DLL Path"=w18:path)  [unwired: 6 in]
  n7 = local write "User Input"(w3) -> ()
  n8 = while {
    tunnel: w18 -> [w49]
    tunnel: w16 -> [w48]
    shift-right: [w41] -> _
    shift-left: FIFOStream_States."Idle" ("State") -> [w50]
    shift-right: [w44] -> _
    shift-left: w28 -> [w43]
    tunnel: w17 -> [w45]
    tunnel: [w46] -> w12
    shift-right: [w40] -> _
    shift-left: _ -> [w39]
    shift-right: [w38] -> _
    shift-left: _ -> [w37]
    stop <- w47 stop-if-true
    n9 = case shown="\"PrepareMeas\"" w50 {
      tunnel: w49 -> [_ w86 w120 w139 _ w221]
      tunnel: w45 -> [w56 w85 w118 w137 _ w223]
      tunnel: w48 -> [_ w87 w119 w138 _ w222]
      tunnel: [w58 FIFOStream_States."TestState" ("State") w112 FIFOStream_States."Analyze" ("State") w177 FIFOStream_States."Idle" ("State")] -> w41
      tunnel: [w56 w72 w123 w124 _ w218] -> w46
      tunnel: [w57 w93 w122 w125 w153 w216] -> w44
      tunnel: w43 -> [w57 _ w122 w136 w153 w217]
      tunnel: [w52 w94 w121 w129 w172 w209] -> w40
      tunnel: w39 -> [w52 _ w121 w129 w171 w209]
      tunnel: [_ _ _ w127 _ _] -> w38
      tunnel: w37 -> [_ _ _ _ w154 _]
      frame "Idle", Default {
        n10 = Select(t=FIFOStream_States."PrepareMeas" ("State"), s="Start Meas", f=FIFOStream_States."Idle" ("State")) -> (s? t:f=w58:T3)
        n11 = Wait (ms)(milliseconds to wait=u32 50) -> ()  [unwired: 1 out]
      }
      frame "PrepareMeas" {
        w68 = FALSE ("Photon Count reached")
        w79 = i32[] []  # FlagEvents
        w88 = u64 0  # TimeLine
        w91 = i16 8192  # FREE_BUF_STREAM
        w63 = T2[] []  # PhotInfo64
        w96 = 0  # Decay
        w99 = T11 {"Valid Photons"=TRUE, "Invalid Photons"=FALSE, "Pixel"=FALSE, "Line"=FALSE, "Frame"=FALSE, "Marker 3"=FALSE}  # What to Read
        # "prepare the upcoming measurement"
        n12 = call "SPC_get_parameters.vi"("Error In"=w85, "Module No"=w87, "DLL Path"=w86) -> ("Error Out"=w67:errorcluster, "Module No"=w66:i16, "DLL Path"=w65:path, "SPCdata"=w84:T9)  [unwired: 5 in]
        n13 = local write "Photon Count reached"(w68) -> ()
        n14 = local write "Col.TimerExpired"(w68) -> ()
        n15 = Unbundle By Name(w84) -> ("collect_time"=w81:sgl)
        n16 = call "SPC_get_fifo_init_vars.vi"("Error In"=w67, "Module No."=w66, "DLL Path"=w65) -> ("Error Out"=w102:errorcluster, "Module No."=w101:i16, "DLL Path"=w103:path, "mt_clock ( 0.1 ns units)"=w64:i32, "Fifo Type"=w60:T5, "stream_type"=w100:i16)  [unwired: 2 in, 1 out]
        "Fifo Type" <- w60
        n17 = Multiply(x="BinningResolution [ms]", y=0.001) -> (x*y=w61:dbl)
        n18 = Divide(x=w81, y=w61) -> (x/y=w80:dbl)
        n19 = Divide(x=w64, y=10.0) -> (x/y=w62:dbl)
        "MT clock [ns]" <- w62
        n20 = property on="MCS TimeLine" class="WFGraph (strict)"("XScale.Multiplier"=w61) -> ()  [unwired: 2 in, 2 out]
        n21 = Multiply(x=w62, y=1e-09) -> (x*y=w77:dbl)
        n22 = Divide(x=w61, y=w77) -> (x/y=w76:dbl)
        n23 = To Long Integer(number=w76) -> (32bit integer=→"MTDivider":i32)
        n24 = Or(x=w91, y=w100) -> (x .or. y?=w92:i16)
        n25 = call "SPC_init_buf_stream.vi"("Start01_offs ( for DPC modules)"=u32 0, "Stream Type"=w92, "MT clock ( 0.1 ns units)"=w64, "FIFO Type"=w60, "Error In"=w102, "What to Read"=w99, "Module No"=w101, "DLL Path"=w103) -> ("Error Out"=w73:errorcluster, "Stream Handle"=w93:i16, "Module No"=w71:i16, "DLL Path"=w70:path)
        "StreamHandle" <- w93
        n26 = Initialize Array(w96, 4096 ("dimension size")) -> (w90:i32[])
        n27 = local write "MCS TimeLine"(u64[] [] ("TimeLine")) -> ()
        n28 = local write "Decay"(i32[] [] ("Decay")) -> ()
        n29 = Initialize Array(w88, w80) -> (w89:u64[])
        n30 = call "SPC_start_measurement.vi"("Error In"=w73, "Module No"=w71, "DLL Path"=w70) -> ("Error Out"=w72:errorcluster)  [unwired: 6 in, 2 out]
        n31 = Bundle("PhotInfo64"=w63, w89, w90, "FlagEvents"=w79) -> (w94:T12)  [unwired: 1 in]
      }
      frame "TestState" {
        # "UserAbort"
        # "Start Measurement and check if ready"
        n32 = call "CheckState.vi"("Error In"=w118, "Module No."=w119, "DLL Path"=w120) -> ("Error Out"=w123:errorcluster, "SPC_StateCluster"=w107:T1)  [unwired: 4 in, 3 out]
        n33 = local write "SPC_StateCluster"(w107) -> ()
        n34 = Unbundle By Name(w107) -> ("MEASURE"=w117:bool, "FEMPTY"=w106:bool, "ARMED"=w108:bool)
        n35 = Not(x=w108) -> (.not. x?=w105:bool)
        n36 = Compound Arithmetic op=AND "data to collect"(w117, invert w106) -> (w116:bool)
        n37 = And(x=w106, y=w105) -> (x .and. y?=→"Col.TimerExpired":bool)
        n38 = Or "finished, pick\nup last data"(x=w116, y=w105) -> (x .or. y?=w109:bool)
        n39 = local read "Start Meas"() -> (w111:bool)
        n40 = Select(t=FIFOStream_States."ReadFIFO2Stream" ("State"), s=w109, f=FIFOStream_States."TestState") -> (s? t:f=w113:T3)
        n41 = Select(t=w113, s=w111, f=FIFOStream_States."Idle") -> (s? t:f=w112:T3)
      }
      frame "ReadFIFO2Stream" {
        w126 = T2[] []  # PhotInfo64
        # "SPC_read_fifo_to_stream,    SPC_get_photons_from_stream"
        n42 = call "SPC_read_fifo_to_stream.vi"("Stream Handle"=w136, "MaxCount"=u32 15000000 ("Count"), "Error In"=w137, "Module No"=w138, "DLL Path"=w139) -> ("Error Out"=w135:errorcluster, "Module No"=w133:i16, "DLL Path"=w134:path, "Stream Handle"=w132:i16, "Count"=→"EventCount":u32)  [unwired: 2 in]
        n43 = while {
          tunnel: w134 -> [w151]
          tunnel: w133 -> [w150]
          tunnel: w132 -> [w149]
          shift-right: [w145] -> w127
          shift-left: w126 -> [w147]
          tunnel: [w144] -> w125
          shift-right: [w140] -> w124
          shift-left: w135 -> [w152]
          stop <- w142 stop-if-true
          # "error code +2 indicates all photons read.\nerror code +1 indicates a stop condition\n                        found. (Not in this scenario)"
          # "read the whole buffered stream in max 1M chunks"
          n44 = call "SPC_get_photons_from_stream.vi"("Stream Handle"=w149, "EventCount"=u32 1000000, "Error In"=w152, "Module No"=w150, "DLL Path"=w151) -> ("Error Out"=w140:errorcluster, "Stream Handle"=w144:i16, "PhotInfo64"=w146:T2[])  [unwired: 1 in, 3 out]
          n45 = Build Array (concatenate)(w147, w146) -> (w145:T2[])
          n46 = Unbundle By Name(w140) -> ("Code"=w143:i32)
          n47 = Greater Than 0?(x=w143) -> (x > 0?=w141:bool)
          n48 = Or(x=w141, y=w140) -> (x .or. y?=w142:bool)
        }
      }
      frame "Analyze" {
        # "Data distribution to graphs"
        n49 = local read "MTDivider"() -> (w164:i32)
        n50 = Unbundle(w171) -> ("PhotInfo64"=w167:T2[], w157:u64[], w156:i32[], "FlagEvents"=w155:i32[])
        n51 = Array Size(array=w167) -> (size(s)=w166:i32)
        n52 = for {
          shift-right: [w192] -> w160
          shift-left: w156 -> [w193]
          tunnel: "Photons to Count" -> [w182]
          tunnel: [w183] -> w168
          shift-right: [w188] -> w162
          shift-left: w157 -> [w191]
          tunnel: w164 -> [w186]
          tunnel: [w181] -> w165 mode=indexing if=w185
          tunnel: w166 -> [w180]
          tunnel: [w179] -> w159
          tunnel: [w178] -> w158 mode=indexing
          tunnel: w154 -> [w178] mode=indexing
          stop <- w183 stop-if-true
          n53 = Unbundle By Name(w178) -> ("mtime"=w187:u64, "micro_time"=w190:u16, "flags"=w194:u16)
          n54 = Increment(x=w180) -> (x+1=w179:i32)
          n55 = Greater Or Equal?(x=w179, y=w182) -> (x >= y?=w183:bool)
          n56 = Equal To 0?(x=w194) -> (x = 0?=w184:bool)
          n57 = Quotient & Remainder(x=w187, y=w186) -> (floor(x/y)=w189:u64)  [unwired: 1 out]
          n58 = Not(x=w184) -> (.not. x?=w185:bool)
          n59 = case shown="True" w184 {
            tunnel: w193 -> [w201 w204]
            tunnel: w190 -> [_ w203]
            tunnel: [w201 w202] -> w192
            frame False {
            }
            frame True {
              # "populate decay curve"
              n60 = in-place {
                n61 = in-place-array #1(w204, w203) -> (w206:i32)
                n62 = Increment(x=w206) -> (x+1=w205:i32)
                n63 = in-place-array #1(w205) -> (w202:i32[])  [unwired: 1 out]
              }
            }
          }
          n64 = case shown="True" w184 {
            tunnel: w191 -> [w195 w198]
            tunnel: w189 -> [_ w197]
            tunnel: [w195 w196] -> w188
            frame False {
            }
            frame True {
              # "bin into timeline"
              n65 = in-place {
                n66 = in-place-array #2(w198, w197) -> (w200:u64)
                n67 = Increment(x=w200) -> (x+1=w199:u64)
                n68 = in-place-array #2(w199) -> (w196:u64[])  [unwired: 1 out]
              }
            }
          }
          n69 = Decrement(x=w179) -> (x-1=w181:i32)
        }
        "Photon Count reached" <- w168
        "PhotonCount" <- w159
        "Decay" <- w160
        "MCS TimeLine" <- w162
        n70 = Build Array (concatenate)(w155, w165) -> (w161:i32[])
        "FlagEvents" <- w161
        n71 = Build Array (concatenate)(w167, w158) -> (w163:T2[])
        "PhotInfo64" <- w163
        n72 = Bundle(w163, w162, w160, w161) -> (w172:cluster{T2[], u64[], i32[], i32[]})  [unwired: 1 in]
        n73 = local read "Col.TimerExpired"() -> (w169:bool)
        n74 = local read "Start Meas"() -> (w173:bool)
        n75 = Compound Arithmetic op=OR(invert w173, w169, w168) -> (w174:bool)
        n76 = Select(t=FIFOStream_States."StopMeas" ("State"), s=w174, f=FIFOStream_States."TestState" ("State")) -> (s? t:f=w177:T3)
      }
      frame "StopMeas" {
        # "at the end close the opened stream"
        # "SPC_stop_measurement should be called even if the measurement was stopped after collection time to set DLL internal variables"
        # "Stop the previous started measurement"
        n77 = call "SPC_stop_measurement.vi"("Error In"=w223, "Module No"=w222, "DLL Path"=w221) -> ("Error Out"=w219:errorcluster, "DLL Path"=w215:path)  [unwired: 6 in, 1 out]
        n78 = local write "Start Meas"(FALSE ("Start Meas")) -> ()
        n79 = Unbundle By Name(w209) -> ("FlagEvents"=w208:i32[], "PhotInfo64"=w207:T2[])
        n80 = call "SPC_close_phot_stream.vi"("Stream Handle"=w217, "Error In"=w219, "DLL Path"=w215) -> ("Error Out"=w218:errorcluster, "Stream Handle"=w216:i16)  [unwired: 6 in, 1 out]
        n81 = Empty Array?(array=w208) -> (empty?=w213:bool)
        n82 = Array Size(array=w207) -> (size(s)=w210:i32)
        n83 = case "point to possible error flags (SPC_FOVFL)" shown="False" w213 {
          tunnel: w208 -> [w224 _]
          tunnel: [T10 {"Text Color"=16777226, "Background Color"=16711680} ("Numeric Text.Text Colors") T10 {"Text Color"=0, "Background Color"=11776947} ("Numeric Text.Text Colors")] -> w212
          tunnel: [w224 w227] -> w211
          tunnel: w210 -> [_ w228]
          frame False {
            # "macro time information after the overrun is not consistent, consider to break the measurement and lower photon's rate"
          }
          frame True {
            n84 = Decrement(x=w228) -> (x-1=w226:i32)
            n85 = Build Array(w226) -> (w227:i32[])
          }
        }
        n86 = property on="PhotInfo64" class="Arr (strict)"("Index Values"=w211) -> ()  [unwired: 2 in, 2 out]
        n87 = property on="flags" class="DigNum (strict)"("NumText.TextColors"=w212) -> ()  [unwired: 2 in, 2 out]
      }
    }
    "State" <- w41
    n88 = Or(x="Stop", y=w46) -> (x .or. y?=w47:bool)
  }
  n89 = while {
    tunnel: w16 -> [w234]
    tunnel: w18 -> [w235]
    tunnel: w17 -> [w236]
    tunnel: [w233] -> w15
    stop <- w232 stop-if-true
    n90 = event shown="[3] \"User Input.tac_limit_high\": Value Change" {
      selector: _ -> [_ _ _ _ _ _ _ _ _ _ _ _ _]
      dyn-events: _ -> [_ _ _ _ _ _ _ _ _ _ _ _ _]
      timeout: 1000 -> [_ _ _ _ _ _ _ _ _ _ _ _ _]
      tunnel: w236 -> [w252 w267 w275 w282 w289 w299 w306 w313 w320 w327 w334 _ _]
      tunnel: [w242 w256 w272 w279 w286 w296 w303 w310 w317 w324 w331 _ _] -> w233
      tunnel: w235 -> [w251 w269 w273 w280 w287 w297 w304 w311 w318 w325 w332 _ _]
      tunnel: w234 -> [w250 w266 w274 w281 w288 w298 w305 w312 w319 w326 w333 _ _]
      event Value Change {
        w253 = T13 8 items=["CFD Limit Low", "CFD Limit High", "CFD Zero Cross Level", "CFD Holdoff", "SYNC Zero Cross Level", "SYNC Freq Divider", "SYNC Holdoff", "SYNC Threshold", "TAC Range", "TAC Gain", "TAC Offset", "TAC Limit Low", "TAC Limit High", "ADC Resolution", "External Latch Delay", "Collect Time", "Display Time", "Repeat Time", "Stop On Time", "Stop On Overflow", "Dither Range", "Count Increment", "Memory Bank", "Dead Time Compensation", "Scan Control", "Routing Mode", "TAC Enable Hold", "Operation Mode", "Scan Size X", "Scan Size Y", "Scan Routing X Bits", "Scan Routing Y Bits", "Scan Polarity", "Scan Flyback", "Scan Borders", "Pixel Time", "Pixel Clock Source", "Scan Line Compression", "External Trigger Condition", "External Pixel Clock Divider", "Rate Counting Time", "Macro Time Clock", "ADD Signal Source", "ADC Zoom", "XY Gain", "Image Size X", "Image Size Y", "Image Routing X Bits", "Image Routing Y Bits", "Master Clock", "ADC Sample Delay", "Detector Type", "X Axis Type", "Channel Enable", "Channel Slope", "Channel Spec_no"] ("SPC parameter ID")
        n91 = event-data() -> ("NewVal"=w249:sgl)  [unwired: 1 in]
        n92 = call "SPC_set_parameter.vi"("SPC parameter ID"=w253, "Parameter Value"=w249, "Error In"=w252, "Module no"=w250, "DLL Path"=w251) -> ("Error Out"=w248:errorcluster, "Module no"=w247:i16, "DLL Path"=w246:path, "Current Parameter Value"=w237:sgl)  [unwired: 3 in]
        n93 = property on="tac_range" class="DigNum (strict)"("Value"=w237) -> ()  [unwired: 2 in, 2 out]
        n94 = call "SPC_get_parameters.vi"("Error In"=w248, "Module No"=w247, "DLL Path"=w246) -> ("Error Out"=w243:errorcluster, "SPCdata"=w244:T9)  [unwired: 5 in, 2 out]
        n95 = Unbundle By Name(w244) -> ("tac_range"=w241:sgl, "tac_gain"=w240:i16)
        n96 = Divide(x=w241, y=w240) -> (x/y=w238:sgl)
        n97 = Divide(x=w238, y=sgl 4096.0) -> (x/y=w239:sgl)
        n98 = property on="Decay" class="WFGraph (strict)"(error in=w243, "XScale.Multiplier"=w239, "XScale.Maximum"=w238) -> (error out=w242:errorcluster)  [unwired: 1 in, 1 out]
      }
      event Value Change {
        w268 = T13 9 items=["CFD Limit Low", "CFD Limit High", "CFD Zero Cross Level", "CFD Holdoff", "SYNC Zero Cross Level", "SYNC Freq Divider", "SYNC Holdoff", "SYNC Threshold", "TAC Range", "TAC Gain", "TAC Offset", "TAC Limit Low", "TAC Limit High", "ADC Resolution", "External Latch Delay", "Collect Time", "Display Time", "Repeat Time", "Stop On Time", "Stop On Overflow", "Dither Range", "Count Increment", "Memory Bank", "Dead Time Compensation", "Scan Control", "Routing Mode", "TAC Enable Hold", "Operation Mode", "Scan Size X", "Scan Size Y", "Scan Routing X Bits", "Scan Routing Y Bits", "Scan Polarity", "Scan Flyback", "Scan Borders", "Pixel Time", "Pixel Clock Source", "Scan Line Compression", "External Trigger Condition", "External Pixel Clock Divider", "Rate Counting Time", "Macro Time Clock", "ADD Signal Source", "ADC Zoom", "XY Gain", "Image Size X", "Image Size Y", "Image Routing X Bits", "Image Routing Y Bits", "Master Clock", "ADC Sample Delay", "Detector Type", "X Axis Type", "Channel Enable", "Channel Slope", "Channel Spec_no"] ("SPC parameter ID")
        n99 = event-data() -> ("NewVal"=w270:i16)  [unwired: 1 in]
        n100 = call "SPC_set_parameter.vi"("SPC parameter ID"=w268, "Parameter Value"=w270, "Error In"=w267, "Module no"=w266, "DLL Path"=w269) -> ("Error Out"=w264:errorcluster, "Module no"=w263:i16, "DLL Path"=w265:path, "Current Parameter Value"=w254:sgl)  [unwired: 3 in]
        n101 = property on="tac_gain" class="DigNum (strict)"("Value"=w254) -> ()  [unwired: 2 in, 2 out]
        n102 = call "SPC_get_parameters.vi"("Error In"=w264, "Module No"=w263, "DLL Path"=w265) -> ("Error Out"=w257:errorcluster, "SPCdata"=w258:T9)  [unwired: 5 in, 2 out]
        n103 = Unbundle By Name(w258) -> ("tac_range"=w261:sgl, "tac_gain"=w260:i16)
        n104 = Divide(x=w261, y=w260) -> (x/y=w255:sgl)
        n105 = Divide(x=w255, y=sgl 4096.0) -> (x/y=w259:sgl)
        n106 = property on="Decay" class="WFGraph (strict)"(error in=w257, "XScale.Multiplier"=w259, "XScale.Maximum"=w255) -> (error out=w256:errorcluster)  [unwired: 1 in, 1 out]
      }
      event Value Change {
        w277 = T13 10 items=["CFD Limit Low", "CFD Limit High", "CFD Zero Cross Level", "CFD Holdoff", "SYNC Zero Cross Level", "SYNC Freq Divider", "SYNC Holdoff", "SYNC Threshold", "TAC Range", "TAC Gain", "TAC Offset", "TAC Limit Low", "TAC Limit High", "ADC Resolution", "External Latch Delay", "Collect Time", "Display Time", "Repeat Time", "Stop On Time", "Stop On Overflow", "Dither Range", "Count Increment", "Memory Bank", "Dead Time Compensation", "Scan Control", "Routing Mode", "TAC Enable Hold", "Operation Mode", "Scan Size X", "Scan Size Y", "Scan Routing X Bits", "Scan Routing Y Bits", "Scan Polarity", "Scan Flyback", "Scan Borders", "Pixel Time", "Pixel Clock Source", "Scan Line Compression", "External Trigger Condition", "External Pixel Clock Divider", "Rate Counting Time", "Macro Time Clock", "ADD Signal Source", "ADC Zoom", "XY Gain", "Image Size X", "Image Size Y", "Image Routing X Bits", "Image Routing Y Bits", "Master Clock", "ADC Sample Delay", "Detector Type", "X Axis Type", "Channel Enable", "Channel Slope", "Channel Spec_no"] ("SPC parameter ID")
        n107 = event-data() -> ("NewVal"=w276:sgl)  [unwired: 1 in]
        n108 = call "SPC_set_parameter.vi"("SPC parameter ID"=w277, "Parameter Value"=w276, "Error In"=w275, "Module no"=w274, "DLL Path"=w273) -> ("Error Out"=w272:errorcluster, "Current Parameter Value"=w271:sgl)  [unwired: 3 in, 2 out]
        n109 = property on="tac_offset" class="DigNum (strict)"("Value"=w271) -> ()  [unwired: 2 in, 2 out]
      }
      event Value Change {
        w284 = T13 12 items=["CFD Limit Low", "CFD Limit High", "CFD Zero Cross Level", "CFD Holdoff", "SYNC Zero Cross Level", "SYNC Freq Divider", "SYNC Holdoff", "SYNC Threshold", "TAC Range", "TAC Gain", "TAC Offset", "TAC Limit Low", "TAC Limit High", "ADC Resolution", "External Latch Delay", "Collect Time", "Display Time", "Repeat Time", "Stop On Time", "Stop On Overflow", "Dither Range", "Count Increment", "Memory Bank", "Dead Time Compensation", "Scan Control", "Routing Mode", "TAC Enable Hold", "Operation Mode", "Scan Size X", "Scan Size Y", "Scan Routing X Bits", "Scan Routing Y Bits", "Scan Polarity", "Scan Flyback", "Scan Borders", "Pixel Time", "Pixel Clock Source", "Scan Line Compression", "External Trigger Condition", "External Pixel Clock Divider", "Rate Counting Time", "Macro Time Clock", "ADD Signal Source", "ADC Zoom", "XY Gain", "Image Size X", "Image Size Y", "Image Routing X Bits", "Image Routing Y Bits", "Master Clock", "ADC Sample Delay", "Detector Type", "X Axis Type", "Channel Enable", "Channel Slope", "Channel Spec_no"] ("SPC parameter ID")
        n110 = event-data() -> ("NewVal"=w283:sgl)  [unwired: 1 in]
        n111 = call "SPC_set_parameter.vi"("SPC parameter ID"=w284, "Parameter Value"=w283, "Error In"=w282, "Module no"=w281, "DLL Path"=w280) -> ("Error Out"=w279:errorcluster, "Current Parameter Value"=w278:sgl)  [unwired: 3 in, 2 out]
        n112 = property on="tac_limit_high" class="DigNum (strict)"("Value"=w278) -> ()  [unwired: 2 in, 2 out]
      }
      event Value Change {
        w290 = T13 11 items=["CFD Limit Low", "CFD Limit High", "CFD Zero Cross Level", "CFD Holdoff", "SYNC Zero Cross Level", "SYNC Freq Divider", "SYNC Holdoff", "SYNC Threshold", "TAC Range", "TAC Gain", "TAC Offset", "TAC Limit Low", "TAC Limit High", "ADC Resolution", "External Latch Delay", "Collect Time", "Display Time", "Repeat Time", "Stop On Time", "Stop On Overflow", "Dither Range", "Count Increment", "Memory Bank", "Dead Time Compensation", "Scan Control", "Routing Mode", "TAC Enable Hold", "Operation Mode", "Scan Size X", "Scan Size Y", "Scan Routing X Bits", "Scan Routing Y Bits", "Scan Polarity", "Scan Flyback", "Scan Borders", "Pixel Time", "Pixel Clock Source", "Scan Line Compression", "External Trigger Condition", "External Pixel Clock Divider", "Rate Counting Time", "Macro Time Clock", "ADD Signal Source", "ADC Zoom", "XY Gain", "Image Size X", "Image Size Y", "Image Routing X Bits", "Image Routing Y Bits", "Master Clock", "ADC Sample Delay", "Detector Type", "X Axis Type", "Channel Enable", "Channel Slope", "Channel Spec_no"] ("SPC parameter ID")
        n113 = event-data() -> ("NewVal"=w291:sgl)  [unwired: 1 in]
        n114 = call "SPC_set_parameter.vi"("SPC parameter ID"=w290, "Parameter Value"=w291, "Error In"=w289, "Module no"=w288, "DLL Path"=w287) -> ("Error Out"=w286:errorcluster, "Current Parameter Value"=w285:sgl)  [unwired: 3 in, 2 out]
        n115 = property on="tac_limit_low" class="DigNum (strict)"("Value"=w285) -> ()  [unwired: 2 in, 2 out]
      }
      event Value Change {
        w301 = T13 15 items=["CFD Limit Low", "CFD Limit High", "CFD Zero Cross Level", "CFD Holdoff", "SYNC Zero Cross Level", "SYNC Freq Divider", "SYNC Holdoff", "SYNC Threshold", "TAC Range", "TAC Gain", "TAC Offset", "TAC Limit Low", "TAC Limit High", "ADC Resolution", "External Latch Delay", "Collect Time", "Display Time", "Repeat Time", "Stop On Time", "Stop On Overflow", "Dither Range", "Count Increment", "Memory Bank", "Dead Time Compensation", "Scan Control", "Routing Mode", "TAC Enable Hold", "Operation Mode", "Scan Size X", "Scan Size Y", "Scan Routing X Bits", "Scan Routing Y Bits", "Scan Polarity", "Scan Flyback", "Scan Borders", "Pixel Time", "Pixel Clock Source", "Scan Line Compression", "External Trigger Condition", "External Pixel Clock Divider", "Rate Counting Time", "Macro Time Clock", "ADD Signal Source", "ADC Zoom", "XY Gain", "Image Size X", "Image Size Y", "Image Routing X Bits", "Image Routing Y Bits", "Master Clock", "ADC Sample Delay", "Detector Type", "X Axis Type", "Channel Enable", "Channel Slope", "Channel Spec_no"] ("SPC parameter ID")
        n116 = event-data() -> ("NewVal"=w300:sgl)  [unwired: 1 in]
        n117 = call "SPC_set_parameter.vi"("SPC parameter ID"=w301, "Parameter Value"=w300, "Error In"=w299, "Module no"=w298, "DLL Path"=w297) -> ("Error Out"=w296:errorcluster, "Current Parameter Value"=w293:sgl)  [unwired: 3 in, 2 out]
        n118 = property on="collect_time" class="DigNum (strict)"("Value"=w293) -> ()  [unwired: 2 in, 2 out]
        n119 = local read "BinningResolution [ms]"() -> (w292:dbl)
        n120 = Multiply(x=w292, y=0.001) -> (x*y=w295:dbl)
        n121 = property on="MCS TimeLine" class="WFGraph (strict)"("XScale.Multiplier"=w295, "XScale.Maximum"=w293) -> ()  [unwired: 2 in, 2 out]
      }
      event Value Change {
        w307 = T13 7 items=["CFD Limit Low", "CFD Limit High", "CFD Zero Cross Level", "CFD Holdoff", "SYNC Zero Cross Level", "SYNC Freq Divider", "SYNC Holdoff", "SYNC Threshold", "TAC Range", "TAC Gain", "TAC Offset", "TAC Limit Low", "TAC Limit High", "ADC Resolution", "External Latch Delay", "Collect Time", "Display Time", "Repeat Time", "Stop On Time", "Stop On Overflow", "Dither Range", "Count Increment", "Memory Bank", "Dead Time Compensation", "Scan Control", "Routing Mode", "TAC Enable Hold", "Operation Mode", "Scan Size X", "Scan Size Y", "Scan Routing X Bits", "Scan Routing Y Bits", "Scan Polarity", "Scan Flyback", "Scan Borders", "Pixel Time", "Pixel Clock Source", "Scan Line Compression", "External Trigger Condition", "External Pixel Clock Divider", "Rate Counting Time", "Macro Time Clock", "ADD Signal Source", "ADC Zoom", "XY Gain", "Image Size X", "Image Size Y", "Image Routing X Bits", "Image Routing Y Bits", "Master Clock", "ADC Sample Delay", "Detector Type", "X Axis Type", "Channel Enable", "Channel Slope", "Channel Spec_no"] ("SPC parameter ID")
        n122 = event-data() -> ("NewVal"=w308:sgl)  [unwired: 1 in]
        n123 = call "SPC_set_parameter.vi"("SPC parameter ID"=w307, "Parameter Value"=w308, "Error In"=w306, "Module no"=w305, "DLL Path"=w304) -> ("Error Out"=w303:errorcluster, "Current Parameter Value"=w302:sgl)  [unwired: 3 in, 2 out]
        n124 = property on="sync_threshold" class="DigNum (strict)"("Value"=w302) -> ()  [unwired: 2 in, 2 out]
      }
      event Value Change {
        w315 = T13 4 items=["CFD Limit Low", "CFD Limit High", "CFD Zero Cross Level", "CFD Holdoff", "SYNC Zero Cross Level", "SYNC Freq Divider", "SYNC Holdoff", "SYNC Threshold", "TAC Range", "TAC Gain", "TAC Offset", "TAC Limit Low", "TAC Limit High", "ADC Resolution", "External Latch Delay", "Collect Time", "Display Time", "Repeat Time", "Stop On Time", "Stop On Overflow", "Dither Range", "Count Increment", "Memory Bank", "Dead Time Compensation", "Scan Control", "Routing Mode", "TAC Enable Hold", "Operation Mode", "Scan Size X", "Scan Size Y", "Scan Routing X Bits", "Scan Routing Y Bits", "Scan Polarity", "Scan Flyback", "Scan Borders", "Pixel Time", "Pixel Clock Source", "Scan Line Compression", "External Trigger Condition", "External Pixel Clock Divider", "Rate Counting Time", "Macro Time Clock", "ADD Signal Source", "ADC Zoom", "XY Gain", "Image Size X", "Image Size Y", "Image Routing X Bits", "Image Routing Y Bits", "Master Clock", "ADC Sample Delay", "Detector Type", "X Axis Type", "Channel Enable", "Channel Slope", "Channel Spec_no"] ("SPC parameter ID")
        n125 = event-data() -> ("NewVal"=w314:sgl)  [unwired: 1 in]
        n126 = call "SPC_set_parameter.vi"("SPC parameter ID"=w315, "Parameter Value"=w314, "Error In"=w313, "Module no"=w312, "DLL Path"=w311) -> ("Error Out"=w310:errorcluster, "Current Parameter Value"=w309:sgl)  [unwired: 3 in, 2 out]
        n127 = property on="sync_zc_level" class="DigNum (strict)"("Value"=w309) -> ()  [unwired: 2 in, 2 out]
      }
      event Value Change {
        w321 = T13 5 items=["CFD Limit Low", "CFD Limit High", "CFD Zero Cross Level", "CFD Holdoff", "SYNC Zero Cross Level", "SYNC Freq Divider", "SYNC Holdoff", "SYNC Threshold", "TAC Range", "TAC Gain", "TAC Offset", "TAC Limit Low", "TAC Limit High", "ADC Resolution", "External Latch Delay", "Collect Time", "Display Time", "Repeat Time", "Stop On Time", "Stop On Overflow", "Dither Range", "Count Increment", "Memory Bank", "Dead Time Compensation", "Scan Control", "Routing Mode", "TAC Enable Hold", "Operation Mode", "Scan Size X", "Scan Size Y", "Scan Routing X Bits", "Scan Routing Y Bits", "Scan Polarity", "Scan Flyback", "Scan Borders", "Pixel Time", "Pixel Clock Source", "Scan Line Compression", "External Trigger Condition", "External Pixel Clock Divider", "Rate Counting Time", "Macro Time Clock", "ADD Signal Source", "ADC Zoom", "XY Gain", "Image Size X", "Image Size Y", "Image Routing X Bits", "Image Routing Y Bits", "Master Clock", "ADC Sample Delay", "Detector Type", "X Axis Type", "Channel Enable", "Channel Slope", "Channel Spec_no"] ("SPC parameter ID")
        n128 = event-data() -> ("NewVal"=w322:i16)  [unwired: 1 in]
        n129 = call "SPC_set_parameter.vi"("SPC parameter ID"=w321, "Parameter Value"=w322, "Error In"=w320, "Module no"=w319, "DLL Path"=w318) -> ("Error Out"=w317:errorcluster, "Current Parameter Value"=w316:sgl)  [unwired: 3 in, 2 out]
        n130 = property on="sync_freq_div" class="Ring (strict)"("Value"=w316) -> ()  [unwired: 2 in, 2 out]
      }
      event Value Change {
        w328 = T13 0 items=["CFD Limit Low", "CFD Limit High", "CFD Zero Cross Level", "CFD Holdoff", "SYNC Zero Cross Level", "SYNC Freq Divider", "SYNC Holdoff", "SYNC Threshold", "TAC Range", "TAC Gain", "TAC Offset", "TAC Limit Low", "TAC Limit High", "ADC Resolution", "External Latch Delay", "Collect Time", "Display Time", "Repeat Time", "Stop On Time", "Stop On Overflow", "Dither Range", "Count Increment", "Memory Bank", "Dead Time Compensation", "Scan Control", "Routing Mode", "TAC Enable Hold", "Operation Mode", "Scan Size X", "Scan Size Y", "Scan Routing X Bits", "Scan Routing Y Bits", "Scan Polarity", "Scan Flyback", "Scan Borders", "Pixel Time", "Pixel Clock Source", "Scan Line Compression", "External Trigger Condition", "External Pixel Clock Divider", "Rate Counting Time", "Macro Time Clock", "ADD Signal Source", "ADC Zoom", "XY Gain", "Image Size X", "Image Size Y", "Image Routing X Bits", "Image Routing Y Bits", "Master Clock", "ADC Sample Delay", "Detector Type", "X Axis Type", "Channel Enable", "Channel Slope", "Channel Spec_no"] ("SPC parameter ID")
        n131 = event-data() -> ("NewVal"=w329:sgl)  [unwired: 1 in]
        n132 = call "SPC_set_parameter.vi"("SPC parameter ID"=w328, "Parameter Value"=w329, "Error In"=w327, "Module no"=w326, "DLL Path"=w325) -> ("Error Out"=w324:errorcluster, "Current Parameter Value"=w323:sgl)  [unwired: 3 in, 2 out]
        n133 = property on="cfd_limit_low" class="DigNum (strict)"("Value"=w323) -> ()  [unwired: 2 in, 2 out]
      }
      event Value Change {
        w335 = T13 2 items=["CFD Limit Low", "CFD Limit High", "CFD Zero Cross Level", "CFD Holdoff", "SYNC Zero Cross Level", "SYNC Freq Divider", "SYNC Holdoff", "SYNC Threshold", "TAC Range", "TAC Gain", "TAC Offset", "TAC Limit Low", "TAC Limit High", "ADC Resolution", "External Latch Delay", "Collect Time", "Display Time", "Repeat Time", "Stop On Time", "Stop On Overflow", "Dither Range", "Count Increment", "Memory Bank", "Dead Time Compensation", "Scan Control", "Routing Mode", "TAC Enable Hold", "Operation Mode", "Scan Size X", "Scan Size Y", "Scan Routing X Bits", "Scan Routing Y Bits", "Scan Polarity", "Scan Flyback", "Scan Borders", "Pixel Time", "Pixel Clock Source", "Scan Line Compression", "External Trigger Condition", "External Pixel Clock Divider", "Rate Counting Time", "Macro Time Clock", "ADD Signal Source", "ADC Zoom", "XY Gain", "Image Size X", "Image Size Y", "Image Routing X Bits", "Image Routing Y Bits", "Master Clock", "ADC Sample Delay", "Detector Type", "X Axis Type", "Channel Enable", "Channel Slope", "Channel Spec_no"] ("SPC parameter ID")
        n134 = event-data() -> ("NewVal"=w336:sgl)  [unwired: 1 in]
        n135 = call "SPC_set_parameter.vi"("SPC parameter ID"=w335, "Parameter Value"=w336, "Error In"=w334, "Module no"=w333, "DLL Path"=w332) -> ("Error Out"=w331:errorcluster, "Current Parameter Value"=w330:sgl)  [unwired: 3 in, 2 out]
        n136 = property on="cfd_zc_level" class="DigNum (strict)"("Value"=w330) -> ()  [unwired: 2 in, 2 out]
      }
      event "BinningResolution [ms]": Value Change {
        n137 = event-data() -> ("NewVal"=w337:dbl)  [unwired: 1 in]
        n138 = property on="collect_time" class="DigNum (strict)"() -> ("Value"=w340:sgl)  [unwired: 2 in, 2 out]
        n139 = Multiply(x=w337, y=0.001) -> (x*y=w338:dbl)
        n140 = property on="MCS TimeLine" class="WFGraph (strict)"("XScale.Multiplier"=w338, "XScale.Maximum"=w340) -> ()  [unwired: 2 in, 2 out]
      }
      event Timeout {
        # "allow for \"Stop\" to go through"
        n141 = event-data() -> ()  [unwired: 1 in, 3 out]
      }
    }
    n142 = local read "Stop"() -> (w231:bool)
    n143 = Or(x=w233, y=w231) -> (x .or. y?=w232:bool)
  }
  n144 = flat-sequence {
    tunnel: [w343] -> w30
    tunnel: w17 -> [w343]
    tunnel: [w342] -> w31
    tunnel: w16 -> [w342]
    tunnel: w18 -> [w341]
    tunnel: [w341] -> w32
    frame #0 {
      # "Wait for \ninitialization\nto finish"
      n145 = Wait (ms)(milliseconds to wait=u32 500) -> ()  [unwired: 1 out]
    }
  }
  n146 = Unbundle By Name(w4) -> ("tac_range"=w10:sgl, "tac_gain"=w9:i16)
  n147 = Divide(x=w10, y=w9) -> (x/y=w7:sgl)
  n148 = Divide(x=w7, y=sgl 4096.0) -> (x/y=w2:sgl)
  n149 = while {
    tunnel: w31 -> [w361]
    shift-right: [w349] -> w26
    shift-left: w32 -> [w363]
    tunnel: w30 -> [w364]
    tunnel: [w350] -> w24
    stop <- w368 stop-if-true
    n150 = local read "StreamHandle"() -> (w357:i16)
    n151 = call "SPC_get_phot_stream_info.vi"("Stream Handle"=w357, "Error In"=w364, "Module No"=w361, "DLL Path"=w363) -> ("Error Out"=w359:errorcluster, "Module No"=w360:i16, "DLL Path"=w362:path, "SPC_PhotStreamInfo"=w356:T14)  [unwired: 3 in, 1 out]
    n152 = Unbundle By Name(w356) -> ("Stream Size"=→"Stream Size":u64, "Current Offset in Stream"=→"Current Offset in Stream":u64, "No of Read Photons"=→"No of Read Photons":u64, "Current Time"=→"Current Time":dbl)
    n153 = call <vilib>:"Clear Errors.vi"("error in (no error)"=w359) -> ("error out"=w358:errorcluster)  [unwired: 5 in, 1 out]
    n154 = Wait (ms)(milliseconds to wait=u32 1000) -> ()  [unwired: 1 out]
    n155 = call "SPC_read_rates.vi"("Error In"=w358, "Module No"=w360, "DLL Path"=w362) -> ("Error Out"=w367:errorcluster, "Module No"=w347:i16, "DLL Path"=w348:path, "SPC_RatesCluster"=→"SPC_RatesCluster":T4)  [unwired: 5 in]
    n156 = local read "Start Meas"() -> (w345:bool)
    n157 = call <vilib>:"Clear Errors.vi"("error in (no error)"=w367, "specific error code to clear (0: all)"=-30) -> ("error out"=w351:errorcluster)  [unwired: 4 in, 1 out]
    n158 = case shown="False" w345 {
      tunnel: w351 -> [w375 w376]
      tunnel: [w374 w376] -> w350
      tunnel: [w373 w377] -> w349
      tunnel: w348 -> [w371 w377]
      tunnel: w347 -> [w370 _]
      frame False {
        n159 = call "CheckState.vi"("Error In"=w375, "Module No."=w370, "DLL Path"=w371) -> ("Error Out"=w374:errorcluster, "SPC_StateCluster"=→"SPC_StateCluster":T1, "DLL Path"=w373:path)  [unwired: 4 in, 2 out]
      }
      frame True {
        # "don't interfere with\nmeasurement loop"
      }
    }
    n160 = local read "Stop"() -> (w366:bool)
    n161 = Or(x=w366, y=w350) -> (x .or. y?=w368:bool)
  }
  n162 = property on="Decay" class="WFGraph (strict)"("XScale.Multiplier"=w2, "XScale.Maximum"=w7) -> ()  [unwired: 2 in, 2 out]
  n163 = case shown="Error" w15 {
    frame No Error {
    }
    frame Error {
      n164 = local write "Stop"(TRUE) -> ()
    }
  }
  n165 = case shown="Error" w24 {
    frame No Error {
    }
    frame Error {
      n166 = local write "Stop"(TRUE) -> ()
    }
  }
  n167 = Merge Errors(w15, w12, w24) -> (w25:errorcluster)
  n168 = case shown="Error" w12 {
    frame No Error {
    }
    frame Error {
      n169 = local write "Stop"(TRUE) -> ()
    }
  }
  n170 = call "SPC_close.vi"("Error In"=w25, "DLL Path"=w26) -> ("Error Out"=w27:errorcluster)  [unwired: 8 in, 1 out]
  n171 = call <vilib>:"Simple Error Handler.vi"("error in (no error)"=w27) -> ("error out"=w6:errorcluster)  [unwired: 4 in, 4 out]
  n172 = flat-sequence {
    tunnel: w6 -> [_]
    frame #0 {
      n173 = local write "Stop"(FALSE) -> ()
    }
  }
